vi "DDSSequence_STPrampv1.vi"(6 "Freqeuncy (MHz)":dbl[][](array[numeric]), 7 "Power":dbl[][](array[numeric]), 9 "Channels":T1(ring)=enum."Both channels", 10 "Duration (ms)":dbl[][](array[numeric])) -> (3 "appended instruction string":string="dds reset\rdcp spi:CFR2=0x1000080\rdcp spi:STP0=0x418937\rdcp wait::BNC_IN_A_RISING\rdcp update:u\rdcp spi:STP0=0x339D00002CCCCCCD\rdcp wait:406h:\rdcp update:u\r\rdcp spi:STP0=0x336400002CDBB1CE\rdcp wait:406h:\rdcp update:u\r\rdcp spi:STP0=0x332A00002CEA96CF\rdcp wait:406h:\rdcp update:u\r\rdcp spi:STP0=0x32F100002CF97BD0\rdcp wait:406h:\rdcp update:u\r\rdcp spi:STP0=0x32B800002D0860D1\rdcp wait:406h:\rdcp update:u\r\rdcp spi:STP0=0x327E00002D1745D1\rdcp wait:406h:\rdcp update:u\r\rdcp spi:STP0=0x324500002D262AD2\rdcp wait:406h:\rdcp update:u\r\rdcp spi:STP0=0x320C00002D350FD3\rdcp wait:406h:\rdcp update:u\r\rdcp spi:STP0=0x31D200002D43F4D4\rdcp wait:406h:\rdcp update:u\r\rdcp spi:STP0=0x319900002D52D9D5\rdcp wait:406h:\rdcp update:u\r\rdcp spi:STP0=0x315F00002D61BED6\rdcp wait:406h:\rdcp update:u\r\rdcp spi:STP0=0x312600002D70A3D7\rdcp wait:406h:\rdcp update:u\r\rdcp spi:STP0=0x30ED00002D7F88D8\rdcp wait:406h:\rdcp update:u\r\rdcp spi:STP0=0x30B300002D8E6DD9\rdcp wait:406h:\rdcp update:u\r\rdcp spi:STP0=0x307A00002D9D52DA\rdcp wait:406h:\rdcp update:u\r\rdcp spi:STP0=0x304100002DAC37DB\rdcp wait:406h:\rdcp update:u\r\rdcp spi:STP0=0x300700002DBB1CDC\rdcp wait:406h:\rdcp update:u\r\rdcp spi:STP0=0x2FCE00002DCA01DD\rdcp wait:406h:\rdcp update:u\r\rdcp spi:STP0=0x2F9500002DD8E6DE\rdcp wait:406h:\rdcp update:u\r\rdcp spi:STP0=0x2F5B00002DE7CBDE\rdcp wait:406h:\rdcp update:u\r\rdcp spi:STP0=0x2F4F00002DF6B0DF\rdcp wait:406h:\rdcp update:u\r\rdcp spi:STP0=0x2F4300002E0595E0\rdcp wait:406h:\rdcp update:u\r\rdcp spi:STP0=0x2F3700002E147AE1\rdcp wait:406h:\rdcp update:u\r\rdcp spi:STP0=0x2F2A00002E235FE2\rdcp wait:406h:\rdcp update:u\r\rdcp spi:STP0=0x2F1E00002E3244E3\rdcp wait:406h:\rdcp update:u\r\rdcp spi:STP0=0x2F1200002E4129E4\rdcp wait:406h:\rdcp update:u\r\rdcp spi:STP0=0x2F0500002E500EE5\rdcp wait:406h:\rdcp update:u\r\rdcp spi:STP0=0x2EF900002E5EF3E6\rdcp wait:406h:\rdcp update:u\r\rdcp spi:STP0=0x2EED00002E6DD8E7\rdcp wait:406h:\rdcp update:u\r\rdcp spi:STP0=0x2EE100002E7CBDE8\rdcp wait:406h:\rdcp update:u\r\rdcp spi:STP0=0x2ED400002E8BA2E9\rdcp wait:406h:\rdcp update:u\r\rdcp spi:STP0=0x2EC800002E9A87EA\rdcp wait:406h:\rdcp update:u\r\rdcp spi:STP0=0x2EBC00002EA96CEB\rdcp wait:406h:\rdcp update:u\r\rdcp spi:STP0=0x2EAF00002EB851EC\rdcp wait:406h:\rdcp update:u\r\rdcp spi:STP0=0x2EA300002EC736EC\rdcp wait:406h:\rdcp update:u\r\rdcp spi:STP0=0x2E9700002ED61BED\rdcp wait:406h:\rdcp update:u\r\rdcp spi:STP0=0x2E8B00002EE500EE\rdcp wait:406h:\rdcp update:u\r\rdcp spi:STP0=0x2E7E00002EF3E5EF\rdcp wait:406h:\rdcp update:u\r\rdcp spi:STP0=0x2E7200002F02CAF0\rdcp wait:406h:\rdcp update:u\r\rdcp spi:STP0=0x2E6600002F11AFF1\rdcp wait:406h:\rdcp update:u\r\rdcp spi:STP0=0x2E5900002F2094F2\rdcp wait:406h:\rdcp update:u\r\rdcp spi:STP0=0x2E4D00002F2F79F3\rdcp wait:406h:\rdcp update:u\r\rdcp spi:STP0=0x2E4100002F3E5EF4\rdcp wait:406h:\rdcp update:u\r\rdcp spi:STP0=0x2E3500002F4D43F5\rdcp wait:406h:\rdcp update:u\r\rdcp spi:STP0=0x2E2800002F5C28F6\rdcp wait:406h:\rdcp update:u\r\rdcp spi:STP0=0x2E1C00002F6B0DF7\rdcp wait:406h:\rdcp update:u\r\rdcp spi:STP0=0x2E1000002F79F2F8\rdcp wait:406h:\rdcp update:u\r\rdcp spi:STP0=0x2E0300002F88D7F9\rdcp wait:406h:\rdcp update:u\r\rdcp spi:STP0=0x2DF700002F97BCF9\rdcp wait:406h:\rdcp update:u\r\rdcp spi:STP0=0x2DEB00002FA6A1FA\rdcp wait:406h:\rdcp update:u\r\rdcp spi:STP0=0x2DDF00002FB586FB\rdcp wait:406h:\rdcp update:u\r\rdcp spi:STP0=0x2DD200002FC46BFC\rdcp wait:406h:\rdcp update:u\r\rdcp spi:STP0=0x2DC600002FD350FD\rdcp wait:406h:\rdcp update:u\r\rdcp spi:STP0=0x2DBA00002FE235FE\rdcp wait:406h:\rdcp update:u\r\rdcp spi:STP0=0x2DAD00002FF11AFF\rdcp wait:406h:\rdcp update:u\r\rdcp spi:STP0=0x2DA1000030000000\rdcp wait:406h:\rdcp update:u\r\rdcp spi:STP0=0x2D950000300EE501\rdcp wait:406h:\rdcp update:u\r\rdcp spi:STP0=0x2D890000301DCA02\rdcp wait:406h:\rdcp update:u\r\rdcp spi:STP0=0x2D7C0000302CAF03\rdcp wait:406h:\rdcp update:u\r\rdcp spi:STP0=0x2D700000303B9404\rdcp wait:406h:\rdcp update:u\r\rdcp spi:STP0=0x2D680000304A7905\rdcp wait:406h:\rdcp update:u\r\rdcp spi:STP0=0x2D60000030595E06\rdcp wait:406h:\rdcp update:u\r\rdcp spi:STP0=0x2D57000030684307\rdcp wait:406h:\rdcp update:u\r\rdcp spi:STP0=0x2D4F000030772807\rdcp wait:406h:\rdcp update:u\r\rdcp spi:STP0=0x2D47000030860D08\rdcp wait:406h:\rdcp update:u\r\rdcp spi:STP0=0x2D3F00003094F209\rdcp wait:406h:\rdcp update:u\r\rdcp spi:STP0=0x2D37000030A3D70A\rdcp wait:406h:\rdcp update:u\r\rdcp spi:STP0=0x2D2E000030B2BC0B\rdcp wait:406h:\rdcp update:u\r\rdcp spi:STP0=0x2D26000030C1A10C\rdcp wait:406h:\rdcp update:u\r\rdcp spi:STP0=0x2D1E000030D0860D\rdcp wait:406h:\rdcp update:u\r\rdcp spi:STP0=0x2D16000030DF6B0E\rdcp wait:406h:\rdcp update:u\r\rdcp spi:STP0=0x2D0E000030EE500F\rdcp wait:406h:\rdcp update:u\r\rdcp spi:STP0=0x2D05000030FD3510\rdcp wait:406h:\rdcp update:u\r\rdcp spi:STP0=0x2CFD0000310C1A11\rdcp wait:406h:\rdcp update:u\r\rdcp spi:STP0=0x2CF50000311AFF12\rdcp wait:406h:\rdcp update:u\r\rdcp spi:STP0=0x2CED00003129E413\rdcp wait:406h:\rdcp update:u\r\rdcp spi:STP0=0x2CE500003138C914\rdcp wait:406h:\rdcp update:u\r\rdcp spi:STP0=0x2CDC00003147AE14\rdcp wait:406h:\rdcp update:u\r\rdcp spi:STP0=0x2CD4000031569315\rdcp wait:406h:\rdcp update:u\r\rdcp spi:STP0=0x2CCC000031657816\rdcp wait:406h:\rdcp update:u\r\rdcp spi:STP0=0x2CC4000031745D17\rdcp wait:406h:\rdcp update:u\r\rdcp spi:STP0=0x2CBC000031834218\rdcp wait:406h:\rdcp update:u\r\rdcp spi:STP0=0x2CB4000031922719\rdcp wait:406h:\rdcp update:u\r\rdcp spi:STP0=0x2CAB000031A10C1A\rdcp wait:406h:\rdcp update:u\r\rdcp spi:STP0=0x2CA3000031AFF11B\rdcp wait:406h:\rdcp update:u\r\rdcp spi:STP0=0x2C9B000031BED61C\rdcp wait:406h:\rdcp update:u\r\rdcp spi:STP0=0x2C93000031CDBB1D\rdcp wait:406h:\rdcp update:u\r\rdcp spi:STP0=0x2C8B000031DCA01E\rdcp wait:406h:\rdcp update:u\r\rdcp spi:STP0=0x2C82000031EB851F\rdcp wait:406h:\rdcp update:u\r\rdcp spi:STP0=0x2C7A000031FA6A20\rdcp wait:406h:\rdcp update:u\r\rdcp spi:STP0=0x2C72000032094F21\rdcp wait:406h:\rdcp update:u\r\rdcp spi:STP0=0x2C6A000032183422\rdcp wait:406h:\rdcp update:u\r\rdcp spi:STP0=0x2C62000032271922\rdcp wait:406h:\rdcp update:u\r\rdcp spi:STP0=0x2C5900003235FE23\rdcp wait:406h:\rdcp update:u\r\rdcp spi:STP0=0x2C5100003244E324\rdcp wait:406h:\rdcp update:u\r\rdcp spi:STP0=0x2C4900003253C825\rdcp wait:406h:\rdcp update:u\r\rdcp spi:STP0=0x2C4100003262AD26\rdcp wait:406h:\rdcp update:u\r\rdcp spi:STP0=0x2C39000032719227\rdcp wait:406h:\rdcp update:u\r\rdcp spi:STP0=0x2C30000032807728\rdcp wait:406h:\rdcp update:u\r\rdcp spi:STP0=0x2C280000328F5C29\rdcp wait:406h:\rdcp update:u\r\rdcp spi:STP0=0x2C1C0000329E412A\rdcp wait:406h:\rdcp update:u\r\rdcp spi:STP0=0x2C10000032AD262B\rdcp wait:406h:\rdcp update:u\r\rdcp spi:STP0=0x2C03000032BC0B2C\rdcp wait:406h:\rdcp update:u\r\rdcp spi:STP0=0x2BF7000032CAF02D\rdcp wait:406h:\rdcp update:u\r\rdcp spi:STP0=0x2BEB000032D9D52E\rdcp wait:406h:\rdcp update:u\r\rdcp spi:STP0=0x2BDF000032E8BA2F\rdcp wait:406h:\rdcp update:u\r\rdcp spi:STP0=0x2BD2000032F79F2F\rdcp wait:406h:\rdcp update:u\r\rdcp spi:STP0=0x2BC6000033068430\rdcp wait:406h:\rdcp update:u\r\rdcp spi:STP0=0x2BBA000033156931\rdcp wait:406h:\rdcp update:u\r\rdcp spi:STP0=0x2BAD000033244E32\rdcp wait:406h:\rdcp update:u\r\rdcp spi:STP0=0x2BA1000033333333\rdcp wait:406h:\rdcp update:u\r\rdcp spi:STP0=0x2B95000033421834\rdcp wait:406h:\rdcp update:u\r\rdcp spi:STP0=0x2B8900003350FD35\rdcp wait:406h:\rdcp update:u\r\rdcp spi:STP0=0x2B7C0000335FE236\rdcp wait:406h:\rdcp update:u\r\rdcp spi:STP0=0x2B700000336EC737\rdcp wait:406h:\rdcp update:u\r\rdcp spi:STP0=0x2B640000337DAC38\rdcp wait:406h:\rdcp update:u\r\rdcp spi:STP0=0x2B570000338C9139\rdcp wait:406h:\rdcp update:u\r\rdcp spi:STP0=0x2B4B0000339B763A\rdcp wait:406h:\rdcp update:u\r\rdcp spi:STP0=0x2B3F000033AA5B3B\rdcp wait:406h:\rdcp update:u\r\rdcp spi:STP0=0x2B33000033B9403C\rdcp wait:406h:\rdcp update:u\r\rdcp spi:STP0=0x2B26000033C8253D\rdcp wait:406h:\rdcp update:u\r\rdcp spi:STP0=0x2B1A000033D70A3D\rdcp wait:406h:\rdcp update:u\r\rdcp spi:STP0=0x2B0E000033E5EF3E\rdcp wait:406h:\rdcp update:u\r\rdcp spi:STP0=0x2B01000033F4D43F\rdcp wait:406h:\rdcp update:u\r\rdcp spi:STP0=0x2AF500003403B940\rdcp wait:406h:\rdcp update:u\r\rdcp spi:STP0=0x2AE9000034129E41\rdcp wait:406h:\rdcp update:u\r\rdcp spi:STP0=0x2ADD000034218342\rdcp wait:406h:\rdcp update:u\r\rdcp spi:STP0=0x2AD0000034306843\rdcp wait:406h:\rdcp update:u\r\rdcp spi:STP0=0x2AC40000343F4D44\rdcp wait:406h:\rdcp update:u\r\rdcp spi:STP0=0x2AB80000344E3245\rdcp wait:406h:\rdcp update:u\r\rdcp spi:STP0=0x2AAB0000345D1746\rdcp wait:406h:\rdcp update:u\r\rdcp spi:STP0=0x2A9F0000346BFC47\rdcp wait:406h:\rdcp update:u\r\rdcp spi:STP0=0x2A930000347AE148\rdcp wait:406h:\rdcp update:u\r\rdcp spi:STP0=0x2A8700003489C649\rdcp wait:406h:\rdcp update:u\r\rdcp spi:STP0=0x2A7A00003498AB4A\rdcp wait:406h:\rdcp update:u\r\rdcp spi:STP0=0x2A6E000034A7904A\rdcp wait:406h:\rdcp update:u\r\rdcp spi:STP0=0x2A62000034B6754B\rdcp wait:406h:\rdcp update:u\r\rdcp spi:STP0=0x2A55000034C55A4C\rdcp wait:406h:\rdcp update:u\r\rdcp spi:STP0=0x2A49000034D43F4D\rdcp wait:406h:\rdcp update:u\r\rdcp spi:STP0=0x2A3D000034E3244E\rdcp wait:406h:\rdcp update:u\r\rdcp spi:STP0=0x2A28000034F2094F\rdcp wait:406h:\rdcp update:u\r\rdcp spi:STP0=0x2A1400003500EE50\rdcp wait:406h:\rdcp update:u\r\rdcp spi:STP0=0x29FF0000350FD351\rdcp wait:406h:\rdcp update:u\r\rdcp spi:STP0=0x29EB0000351EB852\rdcp wait:406h:\rdcp update:u\r\rdcp spi:STP0=0x29D60000352D9D53\rdcp wait:406h:\rdcp update:u\r\rdcp spi:STP0=0x29C20000353C8254\rdcp wait:406h:\rdcp update:u\r\rdcp spi:STP0=0x29AD0000354B6755\rdcp wait:406h:\rdcp update:u\r\rdcp spi:STP0=0x29990000355A4C56\rdcp wait:406h:\rdcp update:u\r\rdcp spi:STP0=0x2984000035693157\rdcp wait:406h:\rdcp update:u\r\rdcp spi:STP0=0x2970000035781658\rdcp wait:406h:\rdcp update:u\r\rdcp spi:STP0=0x295C00003586FB58\rdcp wait:406h:\rdcp update:u\r\rdcp spi:STP0=0x294700003595E059\rdcp wait:406h:\rdcp update:u\r\rdcp spi:STP0=0x2933000035A4C55A\rdcp wait:406h:\rdcp update:u\r\rdcp spi:STP0=0x291E000035B3AA5B\rdcp wait:406h:\rdcp update:u\r\rdcp spi:STP0=0x290A000035C28F5C\rdcp wait:406h:\rdcp update:u\r\rdcp spi:STP0=0x28F5000035D1745D\rdcp wait:406h:\rdcp update:u\r\rdcp spi:STP0=0x28E1000035E0595E\rdcp wait:406h:\rdcp update:u\r\rdcp spi:STP0=0x28CC000035EF3E5F\rdcp wait:406h:\rdcp update:u\r\rdcp spi:STP0=0x28B8000035FE2360\rdcp wait:406h:\rdcp update:u\r\rdcp spi:STP0=0x28A30000360D0861\rdcp wait:406h:\rdcp update:u\r\rdcp spi:STP0=0x288F0000361BED62\rdcp wait:406h:\rdcp update:u\r\rdcp spi:STP0=0x287A0000362AD263\rdcp wait:406h:\rdcp update:u\r\rdcp spi:STP0=0x286600003639B764\rdcp wait:406h:\rdcp update:u\r\rdcp spi:STP0=0x2851000036489C65\rdcp wait:406h:\rdcp update:u\r\rdcp spi:STP0=0x283D000036578165\rdcp wait:406h:\rdcp update:u\r\rdcp spi:STP0=0x2828000036666666\rdcp wait:406h:\rdcp update:u\r\rdcp spi:STP0=0x2814000036754B67\rdcp wait:406h:\rdcp update:u\r\rdcp spi:STP0=0x27FF000036843068\rdcp wait:406h:\rdcp update:u\r\rdcp spi:STP0=0x27EB000036931569\rdcp wait:406h:\rdcp update:u\r\rdcp spi:STP0=0x27D6000036A1FA6A\rdcp wait:406h:\rdcp update:u\r\rdcp spi:STP0=0x27C2000036B0DF6B\rdcp wait:406h:\rdcp update:u\r\rdcp spi:STP0=0x27AD000036BFC46C\rdcp wait:406h:\rdcp update:u\r\rdcp spi:STP0=0x2799000036CEA96D\rdcp wait:406h:\rdcp update:u\r\rdcp spi:STP0=0x2785000036DD8E6E\rdcp wait:406h:\rdcp update:u\r\rdcp spi:STP0=0x2770000036EC736F\rdcp wait:406h:\rdcp update:u\r\rdcp spi:STP0=0x275C000036FB5870\rdcp wait:406h:\rdcp update:u\r\rdcp spi:STP0=0x27470000370A3D71\rdcp wait:406h:\rdcp update:u\r\rdcp spi:STP0=0x2733000037192272\rdcp wait:406h:\rdcp update:u\r\rdcp spi:STP0=0x271E000037280773\rdcp wait:406h:\rdcp update:u\r\rdcp spi:STP0=0x270A00003736EC73\rdcp wait:406h:\rdcp update:u\r\rdcp spi:STP0=0x26FD00003745D174\rdcp wait:406h:\rdcp update:u\r\rdcp spi:STP0=0x26F100003754B675\rdcp wait:406h:\rdcp update:u\r\rdcp spi:STP0=0x26E5000037639B76\rdcp wait:406h:\rdcp update:u\r\rdcp spi:STP0=0x26D8000037728077\rdcp wait:406h:\rdcp update:u\r\rdcp spi:STP0=0x26CC000037816578\rdcp wait:406h:\rdcp update:u\r\rdcp spi:STP0=0x26C0000037904A79\rdcp wait:406h:\rdcp update:u\r\rdcp spi:STP0=0x26B40000379F2F7A\rdcp wait:406h:\rdcp update:u\r\rdcp spi:STP0=0x26A7000037AE147B\rdcp wait:406h:\rdcp update:u\r\rdcp spi:STP0=0x269B000037BCF97C\rdcp wait:406h:\rdcp update:u\r\rdcp spi:STP0=0x268F000037CBDE7D\rdcp wait:406h:\rdcp update:u\r\rdcp spi:STP0=0x2682000037DAC37E\rdcp wait:406h:\rdcp update:u\r\rdcp spi:STP0=0x2676000037E9A87F\rdcp wait:406h:\rdcp update:u\r\rdcp spi:STP0=0x266A000037F88D80\rdcp wait:406h:\rdcp update:u\r\rdcp spi:STP0=0x265E000038077280\rdcp wait:406h:\rdcp update:u\r\rdcp spi:STP0=0x2651000038165781\rdcp wait:406h:\rdcp update:u\r\rdcp spi:STP0=0x2645000038253C82\rdcp wait:406h:\rdcp update:u\r\rdcp spi:STP0=0x2639000038342183\rdcp wait:406h:\rdcp update:u\r\rdcp spi:STP0=0x262C000038430684\rdcp wait:406h:\rdcp update:u\r\rdcp spi:STP0=0x262000003851EB85\rdcp wait:406h:\rdcp update:u\r\rdcp spi:STP0=0x261400003860D086\rdcp wait:406h:\rdcp update:u\r\rdcp spi:STP0=0x26080000386FB587\rdcp wait:406h:\rdcp update:u\r\rdcp spi:STP0=0x25FB0000387E9A88\rdcp wait:406h:\rdcp update:u\r\rdcp spi:STP0=0x25EF0000388D7F89\rdcp wait:406h:\rdcp update:u\r\rdcp spi:STP0=0x25E30000389C648A\rdcp wait:406h:\rdcp update:u\r\rdcp spi:STP0=0x25D6000038AB498B\rdcp wait:406h:\rdcp update:u\r\rdcp spi:STP0=0x25CA000038BA2E8C\rdcp wait:406h:\rdcp update:u\r\rdcp spi:STP0=0x25BE000038C9138D\rdcp wait:406h:\rdcp update:u\r\rdcp spi:STP0=0x25B2000038D7F88D\rdcp wait:406h:\rdcp update:u\r\rdcp spi:STP0=0x25A5000038E6DD8E\rdcp wait:406h:\rdcp update:u\r\rdcp spi:STP0=0x2599000038F5C28F\rdcp wait:406h:\rdcp update:u\r\rdcp spi:STP0=0x258D00003904A790\rdcp wait:406h:\rdcp update:u\r\rdcp spi:STP0=0x2580000039138C91\rdcp wait:406h:\rdcp update:u\r\rdcp spi:STP0=0x2574000039227192\rdcp wait:406h:\rdcp update:u\r\rdcp spi:STP0=0x2568000039315693\rdcp wait:406h:\rdcp update:u\r\rdcp spi:STP0=0x255C000039403B94\rdcp wait:406h:\rdcp update:u\r\rdcp spi:STP0=0x254F0000394F2095\rdcp wait:406h:\rdcp update:u\r\rdcp spi:STP0=0x25430000395E0596\rdcp wait:406h:\rdcp update:u\r\rdcp spi:STP0=0x25370000396CEA97\rdcp wait:406h:\rdcp update:u\r\rdcp spi:STP0=0x252A0000397BCF98\rdcp wait:406h:\rdcp update:u\r\rdcp spi:STP0=0x251E0000398AB499\rdcp wait:406h:\rdcp update:u\r\rdcp spi:STP0=0x251A00003999999A\rdcp wait:406h:\rdcp update:u\r\rdcp spi:STP0=0x2516000039A87E9B\rdcp wait:406h:\rdcp update:u\r\rdcp spi:STP0=0x2512000039B7639B\rdcp wait:406h:\rdcp update:u\r\rdcp spi:STP0=0x250E000039C6489C\rdcp wait:406h:\rdcp update:u\r\rdcp spi:STP0=0x250A000039D52D9D\rdcp wait:406h:\rdcp update:u\r\rdcp spi:STP0=0x2506000039E4129E\rdcp wait:406h:\rdcp update:u\r\rdcp spi:STP0=0x2501000039F2F79F\rdcp wait:406h:\rdcp update:u\r\rdcp spi:STP0=0x24FD00003A01DCA0\rdcp wait:406h:\rdcp update:u\r\rdcp spi:STP0=0x24F900003A10C1A1\rdcp wait:406h:\rdcp update:u\r\rdcp spi:STP0=0x24F500003A1FA6A2\rdcp wait:406h:\rdcp update:u\r\rdcp spi:STP0=0x24F100003A2E8BA3\rdcp wait:406h:\rdcp update:u\r\rdcp spi:STP0=0x24ED00003A3D70A4\rdcp wait:406h:\rdcp update:u\r\rdcp spi:STP0=0x24E900003A4C55A5\rdcp wait:406h:\rdcp update:u\r\rdcp spi:STP0=0x24E500003A5B3AA6\rdcp wait:406h:\rdcp update:u\r\rdcp spi:STP0=0x24E100003A6A1FA7\rdcp wait:406h:\rdcp update:u\r\rdcp spi:STP0=0x24DD00003A7904A8\rdcp wait:406h:\rdcp update:u\r\rdcp spi:STP0=0x24D900003A87E9A8\rdcp wait:406h:\rdcp update:u\r\rdcp spi:STP0=0x24D400003A96CEA9\rdcp wait:406h:\rdcp update:u\r\rdcp spi:STP0=0x24D000003AA5B3AA\rdcp wait:406h:\rdcp update:u\r\rdcp spi:STP0=0x24CC00003AB498AB\rdcp wait:406h:\rdcp update:u\r\rdcp spi:STP0=0x24C800003AC37DAC\rdcp wait:406h:\rdcp update:u\r\rdcp spi:STP0=0x24C400003AD262AD\rdcp wait:406h:\rdcp update:u\r\rdcp spi:STP0=0x24C000003AE147AE\rdcp wait:406h:\rdcp update:u\r\rdcp spi:STP0=0x24BC00003AF02CAF\rdcp wait:406h:\rdcp update:u\r\rdcp spi:STP0=0x24B800003AFF11B0\rdcp wait:406h:\rdcp update:u\r\rdcp spi:STP0=0x24B400003B0DF6B1\rdcp wait:406h:\rdcp update:u\r\rdcp spi:STP0=0x24B000003B1CDBB2\rdcp wait:406h:\rdcp update:u\r\rdcp spi:STP0=0x24AB00003B2BC0B3\rdcp wait:406h:\rdcp update:u\r\rdcp spi:STP0=0x24A700003B3AA5B4\rdcp wait:406h:\rdcp update:u\r\rdcp spi:STP0=0x24A300003B498AB5\rdcp wait:406h:\rdcp update:u\r\rdcp spi:STP0=0x249F00003B586FB6\rdcp wait:406h:\rdcp update:u\r\rdcp spi:STP0=0x249B00003B6754B6\rdcp wait:406h:\rdcp update:u\r\rdcp spi:STP0=0x249700003B7639B7\rdcp wait:406h:\rdcp update:u\r\rdcp spi:STP0=0x249300003B851EB8\rdcp wait:406h:\rdcp update:u\r\rdcp spi:STP0=0x248F00003B9403B9\rdcp wait:406h:\rdcp update:u\r\rdcp spi:STP0=0x248B00003BA2E8BA\rdcp wait:406h:\rdcp update:u\r\rdcp spi:STP0=0x248700003BB1CDBB\rdcp wait:406h:\rdcp update:u\r\rdcp spi:STP0=0x248300003BC0B2BC\rdcp wait:406h:\rdcp update:u\r\rdcp spi:STP0=0x247E00003BCF97BD\rdcp wait:406h:\rdcp update:u\r\rdcp spi:STP0=0x247A00003BDE7CBE\rdcp wait:406h:\rdcp update:u\r\rdcp spi:STP0=0x247E00003BED61BF\rdcp wait:406h:\rdcp update:u\r\rdcp spi:STP0=0x248300003BFC46C0\rdcp wait:406h:\rdcp update:u\r\rdcp spi:STP0=0x248700003C0B2BC1\rdcp wait:406h:\rdcp update:u\r\rdcp spi:STP0=0x248B00003C1A10C2\rdcp wait:406h:\rdcp update:u\r\rdcp spi:STP0=0x248F00003C28F5C3\rdcp wait:406h:\rdcp update:u\r\rdcp spi:STP0=0x249300003C37DAC3\rdcp wait:406h:\rdcp update:u\r\rdcp spi:STP0=0x249700003C46BFC4\rdcp wait:406h:\rdcp update:u\r\rdcp spi:STP0=0x249B00003C55A4C5\rdcp wait:406h:\rdcp update:u\r\rdcp spi:STP0=0x249F00003C6489C6\rdcp wait:406h:\rdcp update:u\r\rdcp spi:STP0=0x24A300003C736EC7\rdcp wait:406h:\rdcp update:u\r\rdcp spi:STP0=0x24A700003C8253C8\rdcp wait:406h:\rdcp update:u\r\rdcp spi:STP0=0x24AB00003C9138C9\rdcp wait:406h:\rdcp update:u\r\rdcp spi:STP0=0x24B000003CA01DCA\rdcp wait:406h:\rdcp update:u\r\rdcp spi:STP0=0x24B400003CAF02CB\rdcp wait:406h:\rdcp update:u\r\rdcp spi:STP0=0x24B800003CBDE7CC\rdcp wait:406h:\rdcp update:u\r\rdcp spi:STP0=0x24BC00003CCCCCCD\rdcp wait:406h:\rdcp update:u\r\rdcp spi:STP0=0x24C000003CDBB1CE\rdcp wait:406h:\rdcp update:u\r\rdcp spi:STP0=0x24C400003CEA96CF\rdcp wait:406h:\rdcp update:u\r\rdcp spi:STP0=0x24C800003CF97BD0\rdcp wait:406h:\rdcp update:u\r\rdcp spi:STP0=0x24CC00003D0860D1\rdcp wait:406h:\rdcp update:u\r\rdcp spi:STP0=0x24D000003D1745D1\rdcp wait:406h:\rdcp update:u\r\rdcp spi:STP0=0x24D400003D262AD2\rdcp wait:406h:\rdcp update:u\r\rdcp spi:STP0=0x24D900003D350FD3\rdcp wait:406h:\rdcp update:u\r\rdcp spi:STP0=0x24DD00003D43F4D4\rdcp wait:406h:\rdcp update:u\r\rdcp spi:STP0=0x24E100003D52D9D5\rdcp wait:406h:\rdcp update:u\r\rdcp spi:STP0=0x24E500003D61BED6\rdcp wait:406h:\rdcp update:u\r\rdcp spi:STP0=0x24E900003D70A3D7\rdcp wait:406h:\rdcp update:u\r\rdcp spi:STP0=0x24ED00003D7F88D8\rdcp wait:406h:\rdcp update:u\r\rdcp spi:STP0=0x24F100003D8E6DD9\rdcp wait:406h:\rdcp update:u\r\rdcp spi:STP0=0x24F500003D9D52DA\rdcp wait:406h:\rdcp update:u\r\rdcp spi:STP0=0x24F900003DAC37DB\rdcp wait:406h:\rdcp update:u\r\rdcp spi:STP0=0x24FD00003DBB1CDC\rdcp wait:406h:\rdcp update:u\r\rdcp spi:STP0=0x250100003DCA01DD\rdcp wait:406h:\rdcp update:u\r\rdcp spi:STP0=0x250600003DD8E6DE\rdcp wait:406h:\rdcp update:u\r\rdcp spi:STP0=0x250A00003DE7CBDE\rdcp wait:406h:\rdcp update:u\r\rdcp spi:STP0=0x250E00003DF6B0DF\rdcp wait:406h:\rdcp update:u\r\rdcp spi:STP0=0x251200003E0595E0\rdcp wait:406h:\rdcp update:u\r\rdcp spi:STP0=0x251600003E147AE1\rdcp wait:406h:\rdcp update:u\r\rdcp spi:STP0=0x251A00003E235FE2\rdcp wait:406h:\rdcp update:u\r\rdcp spi:STP0=0x251E00003E3244E3\rdcp wait:406h:\rdcp update:u\r\rdcp spi:STP0=0x252A00003E4129E4\rdcp wait:406h:\rdcp update:u\r\rdcp spi:STP0=0x253700003E500EE5\rdcp wait:406h:\rdcp update:u\r\rdcp spi:STP0=0x254300003E5EF3E6\rdcp wait:406h:\rdcp update:u\r\rdcp spi:STP0=0x254F00003E6DD8E7\rdcp wait:406h:\rdcp update:u\r\rdcp spi:STP0=0x255C00003E7CBDE8\rdcp wait:406h:\rdcp update:u\r\rdcp spi:STP0=0x256800003E8BA2E9\rdcp wait:406h:\rdcp update:u\r\rdcp spi:STP0=0x257400003E9A87EA\rdcp wait:406h:\rdcp update:u\r\rdcp spi:STP0=0x258000003EA96CEB\rdcp wait:406h:\rdcp update:u\r\rdcp spi:STP0=0x258D00003EB851EC\rdcp wait:406h:\rdcp update:u\r\rdcp spi:STP0=0x259900003EC736EC\rdcp wait:406h:\rdcp update:u\r\rdcp spi:STP0=0x25A500003ED61BED\rdcp wait:406h:\rdcp update:u\r\rdcp spi:STP0=0x25B200003EE500EE\rdcp wait:406h:\rdcp update:u\r\rdcp spi:STP0=0x25BE00003EF3E5EF\rdcp wait:406h:\rdcp update:u\r\rdcp spi:STP0=0x25CA00003F02CAF0\rdcp wait:406h:\rdcp update:u\r\rdcp spi:STP0=0x25D600003F11AFF1\rdcp wait:406h:\rdcp update:u\r\rdcp spi:STP0=0x25E300003F2094F2\rdcp wait:406h:\rdcp update:u\r\rdcp spi:STP0=0x25EF00003F2F79F3\rdcp wait:406h:\rdcp update:u\r\rdcp spi:STP0=0x25FB00003F3E5EF4\rdcp wait:406h:\rdcp update:u\r\rdcp spi:STP0=0x260800003F4D43F5\rdcp wait:406h:\rdcp update:u\r\rdcp spi:STP0=0x261400003F5C28F6\rdcp wait:406h:\rdcp update:u\r\rdcp spi:STP0=0x262000003F6B0DF7\rdcp wait:406h:\rdcp update:u\r\rdcp spi:STP0=0x262C00003F79F2F8\rdcp wait:406h:\rdcp update:u\r\rdcp spi:STP0=0x263900003F88D7F9\rdcp wait:406h:\rdcp update:u\r\rdcp spi:STP0=0x264500003F97BCF9\rdcp wait:406h:\rdcp update:u\r\rdcp spi:STP0=0x265100003FA6A1FA\rdcp wait:406h:\rdcp update:u\r\rdcp spi:STP0=0x265E00003FB586FB\rdcp wait:406h:\rdcp update:u\r\rdcp spi:STP0=0x266A00003FC46BFC\rdcp wait:406h:\rdcp update:u\r\rdcp spi:STP0=0x267600003FD350FD\rdcp wait:406h:\rdcp update:u\r\rdcp spi:STP0=0x268200003FE235FE\rdcp wait:406h:\rdcp update:u\r\rdcp spi:STP0=0x268F00003FF11AFF\rdcp wait:406h:\rdcp update:u\r\rdcp spi:STP0=0x269B000040000000\rdcp wait:406h:\rdcp update:u\r\rdcp spi:STP0=0x26A70000400EE501\rdcp wait:406h:\rdcp update:u\r\rdcp spi:STP0=0x26B40000401DCA02\rdcp wait:406h:\rdcp update:u\r\rdcp spi:STP0=0x26C00000402CAF03\rdcp wait:406h:\rdcp update:u\r\rdcp spi:STP0=0x26CC0000403B9404\rdcp wait:406h:\rdcp update:u\r\rdcp spi:STP0=0x26D80000404A7905\rdcp wait:406h:\rdcp update:u\r\rdcp spi:STP0=0x26E5000040595E06\rdcp wait:406h:\rdcp update:u\r\rdcp spi:STP0=0x26F1000040684307\rdcp wait:406h:\rdcp update:u\r\rdcp spi:STP0=0x26FD000040772807\rdcp wait:406h:\rdcp update:u\r\rdcp spi:STP0=0x270A000040860D08\rdcp wait:406h:\rdcp update:u\r\rdcp spi:STP0=0x271A00004094F209\rdcp wait:406h:\rdcp update:u\r\rdcp spi:STP0=0x272A000040A3D70A\rdcp wait:406h:\rdcp update:u\r\rdcp spi:STP0=0x273B000040B2BC0B\rdcp wait:406h:\rdcp update:u\r\rdcp spi:STP0=0x274B000040C1A10C\rdcp wait:406h:\rdcp update:u\r\rdcp spi:STP0=0x275C000040D0860D\rdcp wait:406h:\rdcp update:u\r\rdcp spi:STP0=0x276C000040DF6B0E\rdcp wait:406h:\rdcp update:u\r\rdcp spi:STP0=0x277C000040EE500F\rdcp wait:406h:\rdcp update:u\r\rdcp spi:STP0=0x278D000040FD3510\rdcp wait:406h:\rdcp update:u\r\rdcp spi:STP0=0x279D0000410C1A11\rdcp wait:406h:\rdcp update:u\r\rdcp spi:STP0=0x27AD0000411AFF12\rdcp wait:406h:\rdcp update:u\r\rdcp spi:STP0=0x27BE00004129E413\rdcp wait:406h:\rdcp update:u\r\rdcp spi:STP0=0x27CE00004138C914\rdcp wait:406h:\rdcp update:u\r\rdcp spi:STP0=0x27DF00004147AE14\rdcp wait:406h:\rdcp update:u\r\rdcp spi:STP0=0x27EF000041569315\rdcp wait:406h:\rdcp update:u\r\rdcp spi:STP0=0x27FF000041657816\rdcp wait:406h:\rdcp update:u\r\rdcp spi:STP0=0x2810000041745D17\rdcp wait:406h:\rdcp update:u\r\rdcp spi:STP0=0x2820000041834218\rdcp wait:406h:\rdcp update:u\r\rdcp spi:STP0=0x2831000041922719\rdcp wait:406h:\rdcp update:u\r\rdcp spi:STP0=0x2841000041A10C1A\rdcp wait:406h:\rdcp update:u\r\rdcp spi:STP0=0x2851000041AFF11B\rdcp wait:406h:\rdcp update:u\r\rdcp spi:STP0=0x2862000041BED61C\rdcp wait:406h:\rdcp update:u\r\rdcp spi:STP0=0x2872000041CDBB1D\rdcp wait:406h:\rdcp update:u\r\rdcp spi:STP0=0x2882000041DCA01E\rdcp wait:406h:\rdcp update:u\r\rdcp spi:STP0=0x2893000041EB851F\rdcp wait:406h:\rdcp update:u\r\rdcp spi:STP0=0x28A3000041FA6A20\rdcp wait:406h:\rdcp update:u\r\rdcp spi:STP0=0x28B4000042094F21\rdcp wait:406h:\rdcp update:u\r\rdcp spi:STP0=0x28C4000042183422\rdcp wait:406h:\rdcp update:u\r\rdcp spi:STP0=0x28D4000042271922\rdcp wait:406h:\rdcp update:u\r\rdcp spi:STP0=0x28E500004235FE23\rdcp wait:406h:\rdcp update:u\r\rdcp spi:STP0=0x28F500004244E324\rdcp wait:406h:\rdcp update:u\r\rdcp spi:STP0=0x290600004253C825\rdcp wait:406h:\rdcp update:u\r\rdcp spi:STP0=0x291600004262AD26\rdcp wait:406h:\rdcp update:u\r\rdcp spi:STP0=0x2926000042719227\rdcp wait:406h:\rdcp update:u\r\rdcp spi:STP0=0x2937000042807728\rdcp wait:406h:\rdcp update:u\r\rdcp spi:STP0=0x29470000428F5C29\rdcp wait:406h:\rdcp update:u\r\rdcp spi:STP0=0x29570000429E412A\rdcp wait:406h:\rdcp update:u\r\rdcp spi:STP0=0x2968000042AD262B\rdcp wait:406h:\rdcp update:u\r\rdcp spi:STP0=0x2978000042BC0B2C\rdcp wait:406h:\rdcp update:u\r\rdcp spi:STP0=0x2989000042CAF02D\rdcp wait:406h:\rdcp update:u\r\rdcp spi:STP0=0x2999000042D9D52E\rdcp wait:406h:\rdcp update:u\r\rdcp spi:STP0=0x29C2000042E8BA2F\rdcp wait:406h:\rdcp update:u\r\rdcp spi:STP0=0x29EB000042F79F2F\rdcp wait:406h:\rdcp update:u\r\rdcp spi:STP0=0x2A14000043068430\rdcp wait:406h:\rdcp update:u\r\rdcp spi:STP0=0x2A3D000043156931\rdcp wait:406h:\rdcp update:u\r\rdcp spi:STP0=0x2A66000043244E32\rdcp wait:406h:\rdcp update:u\r\rdcp spi:STP0=0x2A8F000043333333\rdcp wait:406h:\rdcp update:u\r\rdcp spi:STP0=0x2AB8000043421834\rdcp wait:406h:\rdcp update:u\r\rdcp spi:STP0=0x2AE100004350FD35\rdcp wait:406h:\rdcp update:u\r\rdcp spi:STP0=0x2B0A0000435FE236\rdcp wait:406h:\rdcp update:u\r\rdcp spi:STP0=0x2B330000436EC737\rdcp wait:406h:\rdcp update:u\r\rdcp spi:STP0=0x2B5B0000437DAC38\rdcp wait:406h:\rdcp update:u\r\rdcp spi:STP0=0x2B840000438C9139\rdcp wait:406h:\rdcp update:u\r\rdcp spi:STP0=0x2BAD0000439B763A\rdcp wait:406h:\rdcp update:u\r\rdcp spi:STP0=0x2BD6000043AA5B3B\rdcp wait:406h:\rdcp update:u\r\rdcp spi:STP0=0x2BFF000043B9403C\rdcp wait:406h:\rdcp update:u\r\rdcp spi:STP0=0x2C28000043C8253D\rdcp wait:406h:\rdcp update:u\r\rdcp spi:STP0=0x2C51000043D70A3D\rdcp wait:406h:\rdcp update:u\r\rdcp spi:STP0=0x2C7A000043E5EF3E\rdcp wait:406h:\rdcp update:u\r\rdcp spi:STP0=0x2CA3000043F4D43F\rdcp wait:406h:\rdcp update:u\r\rdcp spi:STP0=0x2CCC00004403B940\rdcp wait:406h:\rdcp update:u\r\rdcp spi:STP0=0x2CF5000044129E41\rdcp wait:406h:\rdcp update:u\r\rdcp spi:STP0=0x2D1E000044218342\rdcp wait:406h:\rdcp update:u\r\rdcp spi:STP0=0x2D47000044306843\rdcp wait:406h:\rdcp update:u\r\rdcp spi:STP0=0x2D700000443F4D44\rdcp wait:406h:\rdcp update:u\r\rdcp spi:STP0=0x2D990000444E3245\rdcp wait:406h:\rdcp update:u\r\rdcp spi:STP0=0x2DC20000445D1746\rdcp wait:406h:\rdcp update:u\r\rdcp spi:STP0=0x2DEB0000446BFC47\rdcp wait:406h:\rdcp update:u\r\rdcp spi:STP0=0x2E140000447AE148\rdcp wait:406h:\rdcp update:u\r\rdcp spi:STP0=0x2E3D00004489C649\rdcp wait:406h:\rdcp update:u\r\rdcp spi:STP0=0x2E6600004498AB4A\rdcp wait:406h:\rdcp update:u\r\rdcp spi:STP0=0x2E8F000044A7904A\rdcp wait:406h:\rdcp update:u\r\rdcp spi:STP0=0x2EB8000044B6754B\rdcp wait:406h:\rdcp update:u\r\rdcp spi:STP0=0x2EE1000044C55A4C\rdcp wait:406h:\rdcp update:u\r\rdcp spi:STP0=0x2F0A000044D43F4D\rdcp wait:406h:\rdcp update:u\r\rdcp spi:STP0=0x2F32000044E3244E\rdcp wait:406h:\rdcp update:u\r\rdcp spi:STP0=0x2F5B000044F2094F\rdcp wait:406h:\rdcp update:u\r\rdcp spi:STP0=0x2F8400004500EE50\rdcp wait:406h:\rdcp update:u\r\rdcp spi:STP0=0x2FAD0000450FD351\rdcp wait:406h:\rdcp update:u\r\rdcp spi:STP0=0x2FD60000451EB852\rdcp wait:406h:\rdcp update:u\r\rdcp spi:STP0=0x2FFF0000452D9D53\rdcp wait:406h:\rdcp update:u\r\rdcp spi:STP0=0x30510000453C8254\rdcp wait:406h:\rdcp update:u\r\rdcp spi:STP0=0x30A30000454B6755\rdcp wait:406h:\rdcp update:u\r\rdcp spi:STP0=0x30F50000455A4C56\rdcp wait:406h:\rdcp update:u\r\rdcp spi:STP0=0x3147000045693157\rdcp wait:406h:\rdcp update:u\r\rdcp spi:STP0=0x3199000045781658\rdcp wait:406h:\rdcp update:u\r\rdcp spi:STP0=0x31EB00004586FB58\rdcp wait:406h:\rdcp update:u\r\rdcp spi:STP0=0x323D00004595E059\rdcp wait:406h:\rdcp update:u\r\rdcp spi:STP0=0x328F000045A4C55A\rdcp wait:406h:\rdcp update:u\r\rdcp spi:STP0=0x32E0000045B3AA5B\rdcp wait:406h:\rdcp update:u\r\rdcp spi:STP0=0x3332000045C28F5C\rdcp wait:406h:\rdcp update:u\r\rdcp spi:STP0=0x3384000045D1745D\rdcp wait:406h:\rdcp update:u\r\rdcp spi:STP0=0x33D6000045E0595E\rdcp wait:406h:\rdcp update:u\r\rdcp spi:STP0=0x3428000045EF3E5F\rdcp wait:406h:\rdcp update:u\r\rdcp spi:STP0=0x347A000045FE2360\rdcp wait:406h:\rdcp update:u\r\rdcp spi:STP0=0x34CC0000460D0861\rdcp wait:406h:\rdcp update:u\r\rdcp spi:STP0=0x351E0000461BED62\rdcp wait:406h:\rdcp update:u\r\rdcp spi:STP0=0x35700000462AD263\rdcp wait:406h:\rdcp update:u\r\rdcp spi:STP0=0x35C200004639B764\rdcp wait:406h:\rdcp update:u\r\rdcp spi:STP0=0x3614000046489C65\rdcp wait:406h:\rdcp update:u\r\rdcp spi:STP0=0x3666000046578165\rdcp wait:406h:\rdcp update:u\r\rdcp spi:STP0=0x2CCCCCCD\rdcp wait:125h:\rdcp update:u\rdcp start\r")   [LabVIEW 2016]
uses:
  <vilib>/DAQmx/create/channels.llb/DAQmx Create Channel (AO-Voltage-Basic).vi
  <resource>/objmgr/daqmx.rc
  <vilib>/DAQmx/write.llb/DAQmx Write (Analog 2D DBL NChan NSamp).vi
  <vilib>/DAQmx/configure/timing.llb/DAQmx Timing (Sample Clock).vi
  <vilib>/DAQmx/configure/trigger.llb/DAQmx Start Trigger (Digital Edge).vi
panel:
  in  "source":tag
  in  "physical channels 2":tag
  in  "physical channels":tag
  in  "appended array 2":dbl[](array[numeric])=[0.85, 0.845, 0.84, 0.835, 0.83, 0.825, 0.82, 0.815, 0.8099999999999999, 0.8049999999999999, 0.8, 0.7949999999999999, 0.79, 0.785, 0.78, 0.775, 0.77, 0.765, 0.76, 0.755, 0.75, 0.7475, 0.745, 0.7425, 0.74, 0.7375, 0.735, 0.7325, 0.73, 0.7275, 0.725, 0.7225, 0.72, 0.7175, 0.715, 0.7125, 0.71, 0.7075, 0.705, 0.7025, 0.7, 0.6975, 0.6950000000000001, 0.6925, 0.6900000000000001, 0.6875, 0.685, 0.6825, 0.68, 0.6775, 0.675, 0.6725, 0.67, 0.6675, 0.665, 0.6625, 0.66, 0.6575, 0.655, 0.6525, 0.65, 0.649, 0.648, 0.647, 0.646, 0.645, 0.644, 0.643, 0.642, 0.641, 0.64, 0.639, 0.638, 0.637, 0.636, 0.635, 0.634, 0.633, 0.632, 0.631, 0.63, 0.629, 0.628, 0.627, 0.626, 0.625, 0.624, 0.623, 0.622, 0.621, 0.62, 0.619, 0.618, 0.617, 0.616, 0.615, 0.614, 0.613, 0.612, 0.611, 0.61, 0.60925, 0.6085, 0.60775, 0.607, 0.60625, 0.6054999999999999, 0.60475, 0.604, 0.60325, 0.6025, 0.60175, 0.601, 0.60025, 0.5994999999999999, 0.59875, 0.598, 0.59725, 0.5965, 0.59575, 0.595, 0.59425, 0.5934999999999999, 0.59275, 0.592, 0.5912499999999999, 0.5905, 0.58975, 0.589, 0.5882499999999999, 0.5874999999999999, 0.58675, 0.586, 0.5852499999999999, 0.5845, 0.58375, 0.583, 0.5822499999999999, 0.5814999999999999, 0.58075, 0.58, 0.57975, 0.5794999999999999, 0.5792499999999999, 0.579, 0.57875, 0.5785, 0.5782499999999999, 0.578, 0.57775, 0.5774999999999999, 0.5772499999999999, 0.577, 0.57675, 0.5765, 0.5762499999999999, 0.576, 0.57575, 0.5754999999999999, 0.5752499999999999, 0.575, 0.57475, 0.5745, 0.5742499999999999, 0.574, 0.57375, 0.5734999999999999, 0.5732499999999999, 0.573, 0.57275, 0.5725, 0.5722499999999999, 0.572, 0.57175, 0.5714999999999999, 0.5712499999999999, 0.571, 0.57075, 0.5705, 0.5702499999999999, 0.57, 0.5702499999999999, 0.5705, 0.57075, 0.571, 0.5712499999999999, 0.5714999999999999, 0.57175, 0.572, 0.5722499999999999, 0.5725, 0.57275, 0.573, 0.5732499999999999, 0.5734999999999999, 0.57375, 0.574, 0.5742499999999999, 0.5745, 0.57475, 0.575, 0.5752499999999999, 0.5754999999999999, 0.57575, 0.576, 0.5762499999999999, 0.5765, 0.57675, 0.577, 0.5772499999999999, 0.5774999999999999, 0.57775, 0.578, 0.5782499999999999, 0.5785, 0.57875, 0.579, 0.5792499999999999, 0.5794999999999999, 0.57975, 0.58, 0.58075, 0.5814999999999999, 0.5822499999999999, 0.583, 0.58375, 0.5845, 0.5852499999999999, 0.586, 0.58675, 0.5874999999999999, 0.5882499999999999, 0.589, 0.58975, 0.5905, 0.5912499999999999, 0.592, 0.59275, 0.5934999999999999, 0.59425, 0.595, 0.59575, 0.5965, 0.59725, 0.598, 0.59875, 0.5994999999999999, 0.60025, 0.601, 0.60175, 0.6025, 0.60325, 0.604, 0.60475, 0.6054999999999999, 0.60625, 0.607, 0.60775, 0.6085, 0.60925, 0.61, 0.61125, 0.6125, 0.61375, 0.615, 0.61625, 0.6174999999999999, 0.61875, 0.62, 0.62125, 0.6225, 0.62375, 0.625, 0.62625, 0.6275, 0.62875, 0.63, 0.63125, 0.6325000000000001, 0.63375, 0.635, 0.63625, 0.6375, 0.63875, 0.64, 0.64125, 0.6425000000000001, 0.64375, 0.645, 0.64625, 0.6475, 0.64875, 0.65, 0.65125, 0.6525000000000001, 0.65375, 0.655, 0.65625, 0.6575, 0.6587500000000001, 0.66, 0.6607500000000001, 0.6615, 0.66225, 0.663, 0.6637500000000001, 0.6645, 0.66525, 0.666, 0.6667500000000001, 0.6675, 0.66825, 0.669, 0.66975, 0.6705, 0.67125, 0.672, 0.67275, 0.6735, 0.67425, 0.675, 0.67575, 0.6765, 0.67725, 0.6779999999999999, 0.67875, 0.6795, 0.68025, 0.6809999999999999, 0.68175, 0.6825, 0.6832499999999999, 0.6839999999999999, 0.68475, 0.6855, 0.6862499999999999, 0.6869999999999999, 0.68775, 0.6885, 0.6892499999999999, 0.69, 0.6904999999999999, 0.691, 0.6915, 0.692, 0.6924999999999999, 0.693, 0.6935, 0.694, 0.6944999999999999, 0.695, 0.6955, 0.696, 0.6964999999999999, 0.697, 0.6975, 0.698, 0.6984999999999999, 0.699, 0.6995, 0.7, 0.7004999999999999, 0.701, 0.7015, 0.702, 0.7024999999999999, 0.703, 0.7035, 0.704, 0.7044999999999999, 0.705, 0.7055, 0.706, 0.7064999999999999, 0.707, 0.7075, 0.708, 0.7084999999999999, 0.709, 0.7095, 0.71, 0.71075, 0.7115, 0.7122499999999999, 0.713, 0.71375, 0.7144999999999999, 0.7152499999999999, 0.716, 0.71675, 0.7175, 0.7182499999999999, 0.719, 0.71975, 0.7204999999999999, 0.72125, 0.722, 0.72275, 0.7235, 0.72425, 0.725, 0.72575, 0.7264999999999999, 0.72725, 0.728, 0.72875, 0.7295, 0.73025, 0.731, 0.73175, 0.7324999999999999, 0.73325, 0.734, 0.73475, 0.7355, 0.73625, 0.737, 0.73775, 0.7384999999999999, 0.73925, 0.74, 0.7435, 0.747, 0.7505, 0.754, 0.7575000000000001, 0.761, 0.7645, 0.768, 0.7715000000000001, 0.775, 0.7785, 0.782, 0.7855000000000001, 0.789, 0.7925, 0.796, 0.7995000000000001, 0.803, 0.8065]
  out "Array":dbl[](array[numeric])=[0.85, 0.845, 0.84, 0.835, 0.83, 0.825, 0.82, 0.815, 0.8099999999999999, 0.8049999999999999, 0.8, 0.7949999999999999, 0.79, 0.785, 0.78, 0.775, 0.77, 0.765, 0.76, 0.755]
  in  "Ramp offset":dbl=-1.0 format="%#_13g"
  in  "End Freq (Hz)":i32=275000000
  in  "Power scaling factor":dbl=0.0015 format="%#_13g"
  out "Freq Step (Hz)":i32=227273
  in  "Time step (ms)":dbl=0.00325 format="%#_13g"
  out "Min DDS setting":dbl=0.6715
  in  "Start Freq (Hz)":i32=175000000
  out "appended array":dbl[][](array[numeric])=[[1.0, 1.002, 1.004, 1.006, 1.008, 1.01, 1.012, 1.014, 1.016, 1.018, 1.02, 1.022, 1.024, 1.026, 1.028, 1.03, 1.032, 1.034, 1.036, 1.038, 1.04, 1.042, 1.044, 1.046, 1.048, 1.05, 1.052, 1.054, 1.056, 1.058, 1.06, 1.062, 1.064, 1.066, 1.068, 1.07, 1.072, 1.074, 1.076, 1.078, 1.08, 1.082, 1.084, 1.086, 1.088, 1.09, 1.092, 1.094, 1.096, 1.098, 1.1, 1.102, 1.104, 1.106, 1.108, 1.11, 1.112, 1.114, 1.116, 1.118, 1.12, 1.1219999999999999, 1.124, 1.126, 1.1280000000000001, 1.13, 1.1320000000000001, 1.134, 1.1360000000000001, 1.138, 1.1400000000000001, 1.142, 1.1440000000000001, 1.146, 1.148, 1.15, 1.152, 1.154, 1.156, 1.158, 1.16, 1.162, 1.164, 1.166, 1.168, 1.17, 1.172, 1.174, 1.176, 1.178, 1.18, 1.182, 1.184, 1.186, 1.188, 1.19, 1.192, 1.194, 1.196, 1.198, 1.2, 1.2, 1.2, 1.2, 1.2, 1.2, 1.2, 1.2, 1.2, 1.2, 1.2, 1.2, 1.2, 1.2, 1.2, 1.2, 1.2, 1.2, 1.2, 1.2, 1.2, 1.2, 1.2, 1.2, 1.2, 1.2, 1.2, 1.2, 1.2, 1.2, 1.2, 1.2, 1.2, 1.2, 1.2, 1.2, 1.2, 1.2, 1.2, 1.2, 1.2, 1.2, 1.2, 1.2, 1.2, 1.2, 1.2, 1.2, 1.2, 1.2, 1.2, 1.2, 1.198, 1.196, 1.194, 1.192, 1.19, 1.188, 1.186, 1.184, 1.182, 1.18, 1.178, 1.176, 1.174, 1.172, 1.17, 1.168, 1.166, 1.164, 1.162, 1.16, 1.158, 1.156, 1.154, 1.152, 1.15, 1.148, 1.146, 1.1440000000000001, 1.142, 1.1400000000000001, 1.138, 1.1360000000000001, 1.134, 1.1320000000000001, 1.13, 1.1280000000000001, 1.126, 1.124, 1.1219999999999999, 1.12, 1.118, 1.116, 1.114, 1.112, 1.11, 1.108, 1.106, 1.104, 1.102, 1.1, 1.098, 1.096, 1.094, 1.092, 1.09, 1.088, 1.086, 1.084, 1.082, 1.08, 1.078, 1.076, 1.074, 1.072, 1.07, 1.068, 1.066, 1.064, 1.062, 1.06, 1.058, 1.056, 1.054, 1.052, 1.05, 1.048, 1.046, 1.044, 1.042, 1.04, 1.038, 1.036, 1.034, 1.032, 1.03, 1.028, 1.026, 1.024, 1.022, 1.02, 1.018, 1.016, 1.014, 1.012, 1.01, 1.008, 1.006, 1.004, 1.002, 1.0], [1.0, 1.002, 1.004, 1.006, 1.008, 1.01, 1.012, 1.014, 1.016, 1.018, 1.02, 1.022, 1.024, 1.026, 1.028, 1.03, 1.032, 1.034, 1.036, 1.038, 1.04, 1.042, 1.044, 1.046, 1.048, 1.05, 1.052, 1.054, 1.056, 1.058, 1.06, 1.062, 1.064, 1.066, 1.068, 1.07, 1.072, 1.074, 1.076, 1.078, 1.08, 1.082, 1.084, 1.086, 1.088, 1.09, 1.092, 1.094, 1.096, 1.098, 1.1, 1.102, 1.104, 1.106, 1.108, 1.11, 1.112, 1.114, 1.116, 1.118, 1.12, 1.1219999999999999, 1.124, 1.126, 1.1280000000000001, 1.13, 1.1320000000000001, 1.134, 1.1360000000000001, 1.138, 1.1400000000000001, 1.142, 1.1440000000000001, 1.146, 1.148, 1.15, 1.152, 1.154, 1.156, 1.158, 1.16, 1.162, 1.164, 1.166, 1.168, 1.17, 1.172, 1.174, 1.176, 1.178, 1.18, 1.182, 1.184, 1.186, 1.188, 1.19, 1.192, 1.194, 1.196, 1.198, 1.2, 1.2, 1.2, 1.2, 1.2, 1.2, 1.2, 1.2, 1.2, 1.2, 1.2, 1.2, 1.2, 1.2, 1.2, 1.2, 1.2, 1.2, 1.2, 1.2, 1.2, 1.2, 1.2, 1.2, 1.2, 1.2, 1.2, 1.2, 1.2, 1.2, 1.2, 1.2, 1.2, 1.2, 1.2, 1.2, 1.2, 1.2, 1.2, 1.2, 1.2, 1.2, 1.2, 1.2, 1.2, 1.2, 1.2, 1.2, 1.2, 1.2, 1.2, 1.2, 1.198, 1.196, 1.194, 1.192, 1.19, 1.188, 1.186, 1.184, 1.182, 1.18, 1.178, 1.176, 1.174, 1.172, 1.17, 1.168, 1.166, 1.164, 1.162, 1.16, 1.158, 1.156, 1.154, 1.152, 1.15, 1.148, 1.146, 1.1440000000000001, 1.142, 1.1400000000000001, 1.138, 1.1360000000000001, 1.134, 1.1320000000000001, 1.13, 1.1280000000000001, 1.126, 1.124, 1.1219999999999999, 1.12, 1.118, 1.116, 1.114, 1.112, 1.11, 1.108, 1.106, 1.104, 1.102, 1.1, 1.098, 1.096, 1.094, 1.092, 1.09, 1.088, 1.086, 1.084, 1.082, 1.08, 1.078, 1.076, 1.074, 1.072, 1.07, 1.068, 1.066, 1.064, 1.062, 1.06, 1.058, 1.056, 1.054, 1.052, 1.05, 1.048, 1.046, 1.044, 1.042, 1.04, 1.038, 1.036, 1.034, 1.032, 1.03, 1.028, 1.026, 1.024, 1.022, 1.02, 1.018, 1.016, 1.014, 1.012, 1.01, 1.008, 1.006, 1.004, 1.002, 1.0]]
  in  "Plateau duration (ms)":dbl=1.0
  in  "Ramp duration (ms)":dbl=2.0
  in  "No of samples in ramp":dbl=100.0
  in  "Ramp Amplitude (V)}":dbl=0.2
  in  "error in":errorcluster
  out "Array 2":i32[](array[numeric])=[175000000, 175227273, 175454545, 175681818, 175909091, 176136364, 176363636, 176590909, 176818182, 177045455, 177272727, 177500000, 177727273, 177954545, 178181818, 178409091, 178636364, 178863636, 179090909, 179318182, 179545455, 179772727, 180000000, 180227273, 180454545, 180681818, 180909091, 181136364, 181363636, 181590909, 181818182, 182045455, 182272727, 182500000, 182727273, 182954545, 183181818, 183409091, 183636364, 183863636, 184090909, 184318182, 184545455, 184772727, 185000000, 185227273, 185454545, 185681818, 185909091, 186136364, 186363636, 186590909, 186818182, 187045455, 187272727, 187500000, 187727273, 187954545, 188181818, 188409091, 188636364, 188863636, 189090909, 189318182, 189545455, 189772727, 190000000, 190227273, 190454545, 190681818, 190909091, 191136364, 191363636, 191590909, 191818182, 192045455, 192272727, 192500000, 192727273, 192954545, 193181818, 193409091, 193636364, 193863636, 194090909, 194318182, 194545455, 194772727, 195000000, 195227273, 195454545, 195681818, 195909091, 196136364, 196363636, 196590909, 196818182, 197045455, 197272727, 197500000, 197727273, 197954545, 198181818, 198409091, 198636364, 198863636, 199090909, 199318182, 199545455, 199772727, 200000000, 200227273, 200454545, 200681818, 200909091, 201136364, 201363636, 201590909, 201818182, 202045455, 202272727, 202500000, 202727273, 202954545, 203181818, 203409091, 203636364, 203863636, 204090909, 204318182, 204545455, 204772727, 205000000, 205227273, 205454545, 205681818, 205909091, 206136364, 206363636, 206590909, 206818182, 207045455, 207272727, 207500000, 207727273, 207954545, 208181818, 208409091, 208636364, 208863636, 209090909, 209318182, 209545455, 209772727, 210000000, 210227273, 210454545, 210681818, 210909091, 211136364, 211363636, 211590909, 211818182, 212045455, 212272727, 212500000, 212727273, 212954545, 213181818, 213409091, 213636364, 213863636, 214090909, 214318182, 214545455, 214772727, 215000000, 215227273, 215454545, 215681818, 215909091, 216136364, 216363636, 216590909, 216818182, 217045455, 217272727, 217500000, 217727273, 217954545, 218181818, 218409091, 218636364, 218863636, 219090909, 219318182, 219545455, 219772727, 220000000, 220227273, 220454545, 220681818, 220909091, 221136364, 221363636, 221590909, 221818182, 222045455, 222272727, 222500000, 222727273, 222954545, 223181818, 223409091, 223636364, 223863636, 224090909, 224318182, 224545455, 224772727, 225000000, 225227273, 225454545, 225681818, 225909091, 226136364, 226363636, 226590909, 226818182, 227045455, 227272727, 227500000, 227727273, 227954545, 228181818, 228409091, 228636364, 228863636, 229090909, 229318182, 229545455, 229772727, 230000000, 230227273, 230454545, 230681818, 230909091, 231136364, 231363636, 231590909, 231818182, 232045455, 232272727, 232500000, 232727273, 232954545, 233181818, 233409091, 233636364, 233863636, 234090909, 234318182, 234545455, 234772727, 235000000, 235227273, 235454545, 235681818, 235909091, 236136364, 236363636, 236590909, 236818182, 237045455, 237272727, 237500000, 237727273, 237954545, 238181818, 238409091, 238636364, 238863636, 239090909, 239318182, 239545455, 239772727, 240000000, 240227273, 240454545, 240681818, 240909091, 241136364, 241363636, 241590909, 241818182, 242045455, 242272727, 242500000, 242727273, 242954545, 243181818, 243409091, 243636364, 243863636, 244090909, 244318182, 244545455, 244772727, 245000000, 245227273, 245454545, 245681818, 245909091, 246136364, 246363636, 246590909, 246818182, 247045455, 247272727, 247500000, 247727273, 247954545, 248181818, 248409091, 248636364, 248863636, 249090909, 249318182, 249545455, 249772727, 250000000, 250227273, 250454545, 250681818, 250909091, 251136364, 251363636, 251590909, 251818182, 252045455, 252272727, 252500000, 252727273, 252954545, 253181818, 253409091, 253636364, 253863636, 254090909, 254318182, 254545455, 254772727, 255000000, 255227273, 255454545, 255681818, 255909091, 256136364, 256363636, 256590909, 256818182, 257045455, 257272727, 257500000, 257727273, 257954545, 258181818, 258409091, 258636364, 258863636, 259090909, 259318182, 259545455, 259772727, 260000000, 260227273, 260454545, 260681818, 260909091, 261136364, 261363636, 261590909, 261818182, 262045455, 262272727, 262500000, 262727273, 262954545, 263181818, 263409091, 263636364, 263863636, 264090909, 264318182, 264545455, 264772727, 265000000, 265227273, 265454545, 265681818, 265909091, 266136364, 266363636, 266590909, 266818182, 267045455, 267272727, 267500000, 267727273, 267954545, 268181818, 268409091, 268636364, 268863636, 269090909, 269318182, 269545455, 269772727, 270000000, 270227273, 270454545, 270681818, 270909091, 271136364, 271363636, 271590909, 271818182, 272045455, 272272727, 272500000, 272727273, 272954545, 273181818, 273409091, 273636364, 273863636, 274090909, 274318182, 274545455, 274772727]
  out "return count":u32=26996
  out "error out":errorcluster={"status"=TRUE, "code"=-1073807339, "source"="VISA Read in DDSSequence_STPrampv1.vi"}
  out "read buffer":string
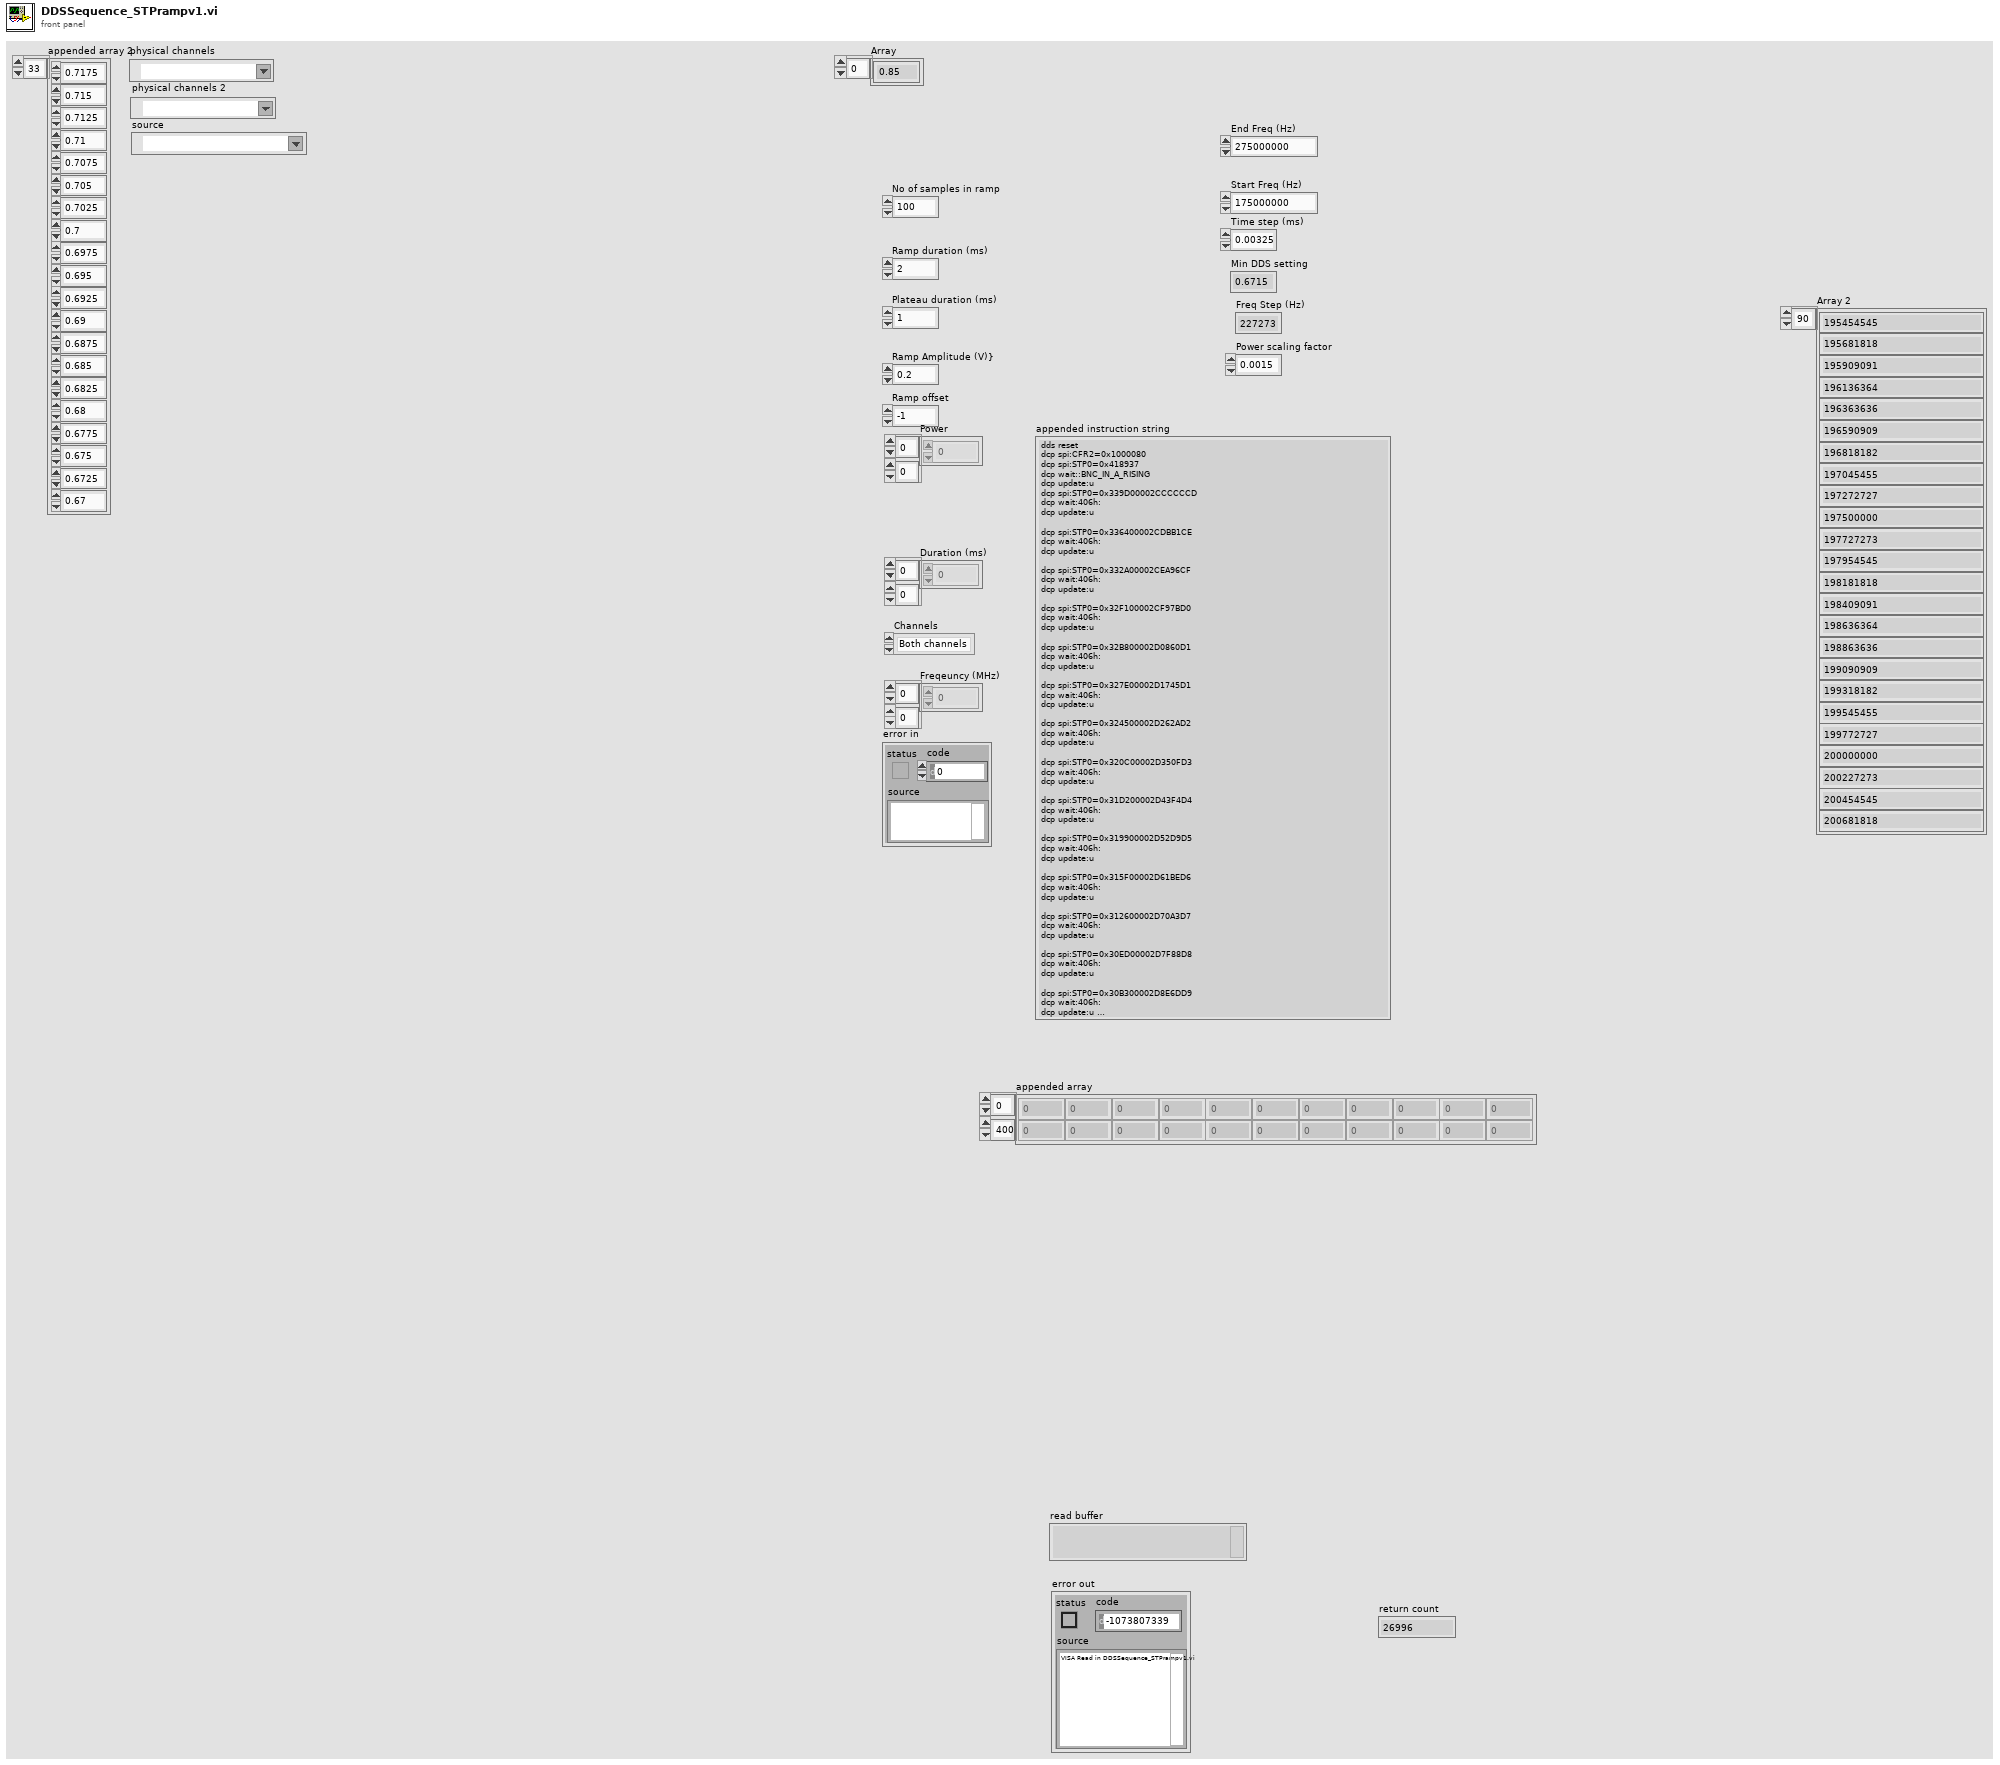
[diagram p1: front panel]
types:
  T1 = enum32{"Channel 0", "Channel 1", "Both channels"}
  T2 = enum32{"O_RAMP_SWP_OVR", "RAM_SWP_OVR", "O_DROVER", "DROVER", "O_SPI_FIFO_EV1", "SPI_FIFO_EV1", "O_SPI_FIFO_EV0", "SPI_FIFO_EV0", "O_SPI_FIFO_FLUSHED", "SPI_FIFO_FLUSHED", "BNC_IN_B_LEVEL", "BNC_IN_B_FALLING", "BNC_IN_B_RISING", "BNC_IN_A_LEVEL", "BNC_IN_A_FALLING", "BNC_IN_A_RISING", "ALL_SPI_FIFOS_FLUSHED", "NONE"}
  T3 = cluster{"Enable ASF from STP (F)":bool, "Digital ramp enable (F)":bool, "Digital ramp no-dwell high (F)":bool, "Digital ramp no-dwell low (F)":bool, "Matched latency enable (T)":bool, "Parallel data port enable (F)":bool}
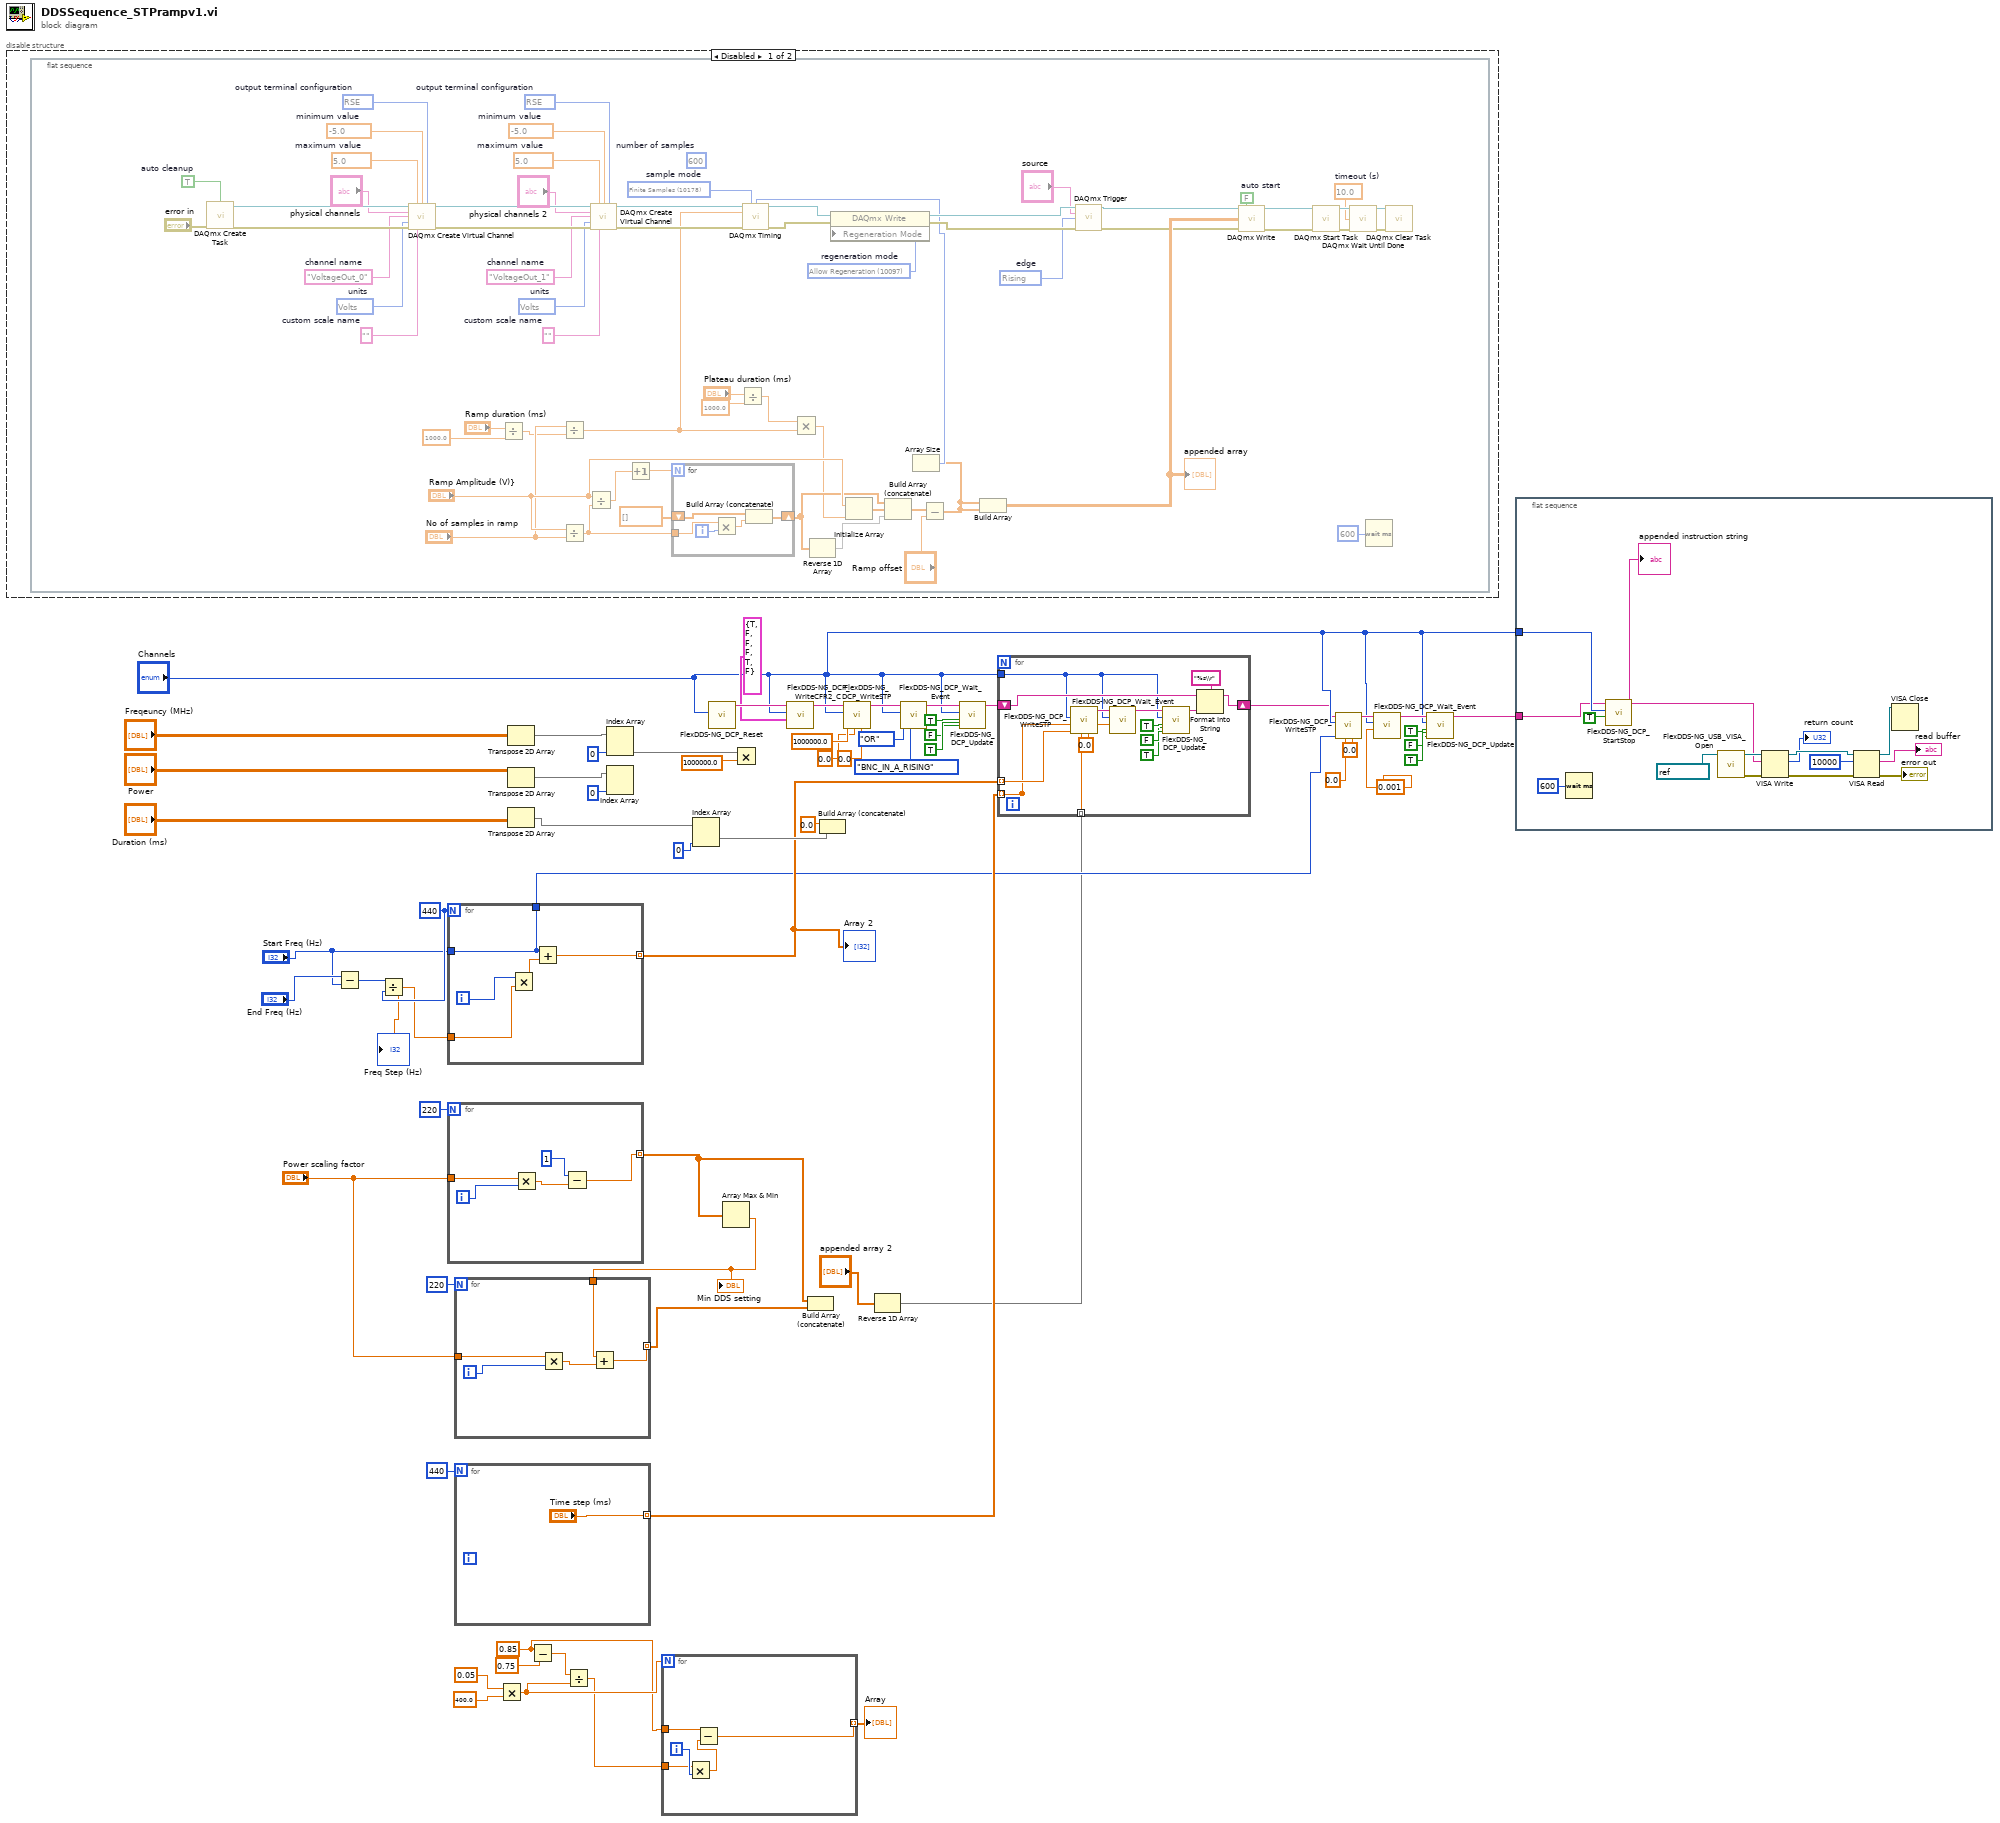
[diagram p0: block diagram]
diagram:
  w5 = 0.85 ("x")
  w14 = 440
  n1 = disable-structure shown="Disabled" {
    frame Disabled {
      n2 = flat-sequence {
        frame #0 {
          w92 = 10280 items=["Rising"=10280, "Falling"=10171]  # edge
          w94 = 10097 items=["Allow Regeneration"=10097, "Do Not Allow Regeneration"=10158]  # regeneration mode
          w97 = 10178 items=["Finite Samples"=10178, "Continuous Samples"=10123, "Hardware Timed Single Point"=12522]  # sample mode
          (unwired) 600  # number of samples
          w100 = 10083 items=["Default"=-1, "RSE"=10083, "Differential"=10106, "Pseudodifferential"=12529]  # output terminal configuration
          w101 = 10348 items=["Volts"=10348, "From Custom Scale"=10065]  # units
          w102 = "VoltageOut_1"  # channel name
          w104 = ""  # custom scale name
          w105 = -5.0  # minimum value
          w106 = 5.0  # maximum value
          w108 = 10083 items=["Default"=-1, "RSE"=10083, "Differential"=10106, "Pseudodifferential"=12529]  # output terminal configuration
          w109 = 10348 items=["Volts"=10348, "From Custom Scale"=10065]  # units
          w110 = "VoltageOut_0"  # channel name
          w112 = ""  # custom scale name
          w113 = -5.0  # minimum value
          w114 = 5.0  # maximum value
          w116 = TRUE  # auto cleanup
          w122 = 10.0  # timeout (s)
          w126 = FALSE  # auto start
          n3 = call <vilib>:"DAQmx Create Task.vi"("auto cleanup"=w116, "error in"="error in") -> ("task out"=w115:refnum<k21>, "error out"=w117:errorcluster)  [unwired: 12 in]
          n4 = call-poly <vilib>:"DAQmx Create Virtual Channel.vi"("task in"=w115, "maximum value"=w114, "minimum value"=w113, "output terminal configuration"=w108, "physical channels"="physical channels", "name to assign"=w110, "units"=w109, "error in"=w117, "custom scale name"=w112) -> ("task out"=w107:refnum<k21>, "error out"=w111:errorcluster)  [unwired: 5 in]
          n5 = Divide(x="Ramp duration (ms)", y=1000.0) -> (x/y=w79:dbl)
          n6 = Divide(x="No of samples in ramp", y=w79) -> (x/y=w74:dbl)
          n7 = Divide(x="Ramp Amplitude (V)}", y="No of samples in ramp") -> (x/y=w90:dbl)
          n8 = Divide(x="Ramp Amplitude (V)}", y=w90) -> (x/y=w89:dbl)
          n9 = call-poly <vilib>:"DAQmx Create Virtual Channel.vi"("task in"=w107, "maximum value"=w106, "minimum value"=w105, "output terminal configuration"=w100, "physical channels"="physical channels 2", "name to assign"=w102, "units"=w101, "error in"=w111, "custom scale name"=w104) -> ("task out"=w98:refnum<k21>, "error out"=w103:errorcluster)  [unwired: 5 in]
          n10 = Increment(x=w89) -> (x+1=w88:dbl)
          n11 = for {
            N: w88 -> [_]
            shift-right: [w129] -> w86
            shift-left: dbl[] [] -> [w128]
            tunnel: w90 -> [w127]
            i -> [w131]
            n12 = Multiply(x=w127, y=w131) -> (x*y=w130:dbl)
            n13 = Build Array (concatenate)(w128, w130) -> (w129:dbl[])
          }
          n14 = Divide(x="Plateau duration (ms)", y=1000.0) -> (x/y=w73:dbl)
          n15 = Multiply(x=w73, y=w74) -> (x*y=w72:dbl)
          n16 = Reverse 1D Array(array=w86) -> (reversed array=w84:dbl[])
          n17 = Initialize Array("Ramp Amplitude (V)}", w72) -> (w85:dbl[])
          n18 = Build Array (concatenate)(w86, w85, w84) -> (w69:dbl[])
          n19 = Subtract(x=w69, y="Ramp offset") -> (x-y=w68:dbl[])
          n20 = Array Size(array=w68) -> (size(s)=w71:i32)
          n21 = call-poly <vilib>:"DAQmx Timing.vi"("task/channels in"=w98, "sample mode"=w97, "samples per channel"=w71, "rate"=w74, "error in"=w103) -> ("task out"=w96:refnum<k21>, "error out"=w99:errorcluster)  [unwired: 9 in]
          n22 = property class="DAQmx Write"(reference=w96, error in=w99, "Regeneration Mode"=w94) -> (reference out=w93:refnum<k21>, error out=w95:errorcluster)
          n23 = Build Array(w68, w68) -> (w83:dbl[][])
          "appended array" <- w83
          n24 = call-poly <vilib>:"DAQmx Trigger.vi"("task/channels in"=w93, "source"="source", "edge"=w92, "error in"=w95) -> ("task out"=w78:refnum<k21>, "error out"=w77:errorcluster)  [unwired: 10 in]
          n25 = call-poly <vilib>:"DAQmx Write.vi"("task/channels in"=w78, "auto start"=w126, "data"=w83, "error in"=w77) -> ("task out"=w121:refnum<k21>, "error out"=w120:errorcluster)  [unwired: 9 in, 1 out]
          n26 = call <vilib>:"DAQmx Start Task.vi"("task/channels in"=w121, "error in"=w120) -> ("task out"=w125:refnum<k21>, "error out"=w124:errorcluster)  [unwired: 12 in]
          n27 = call <vilib>:"DAQmx Wait Until Done.vi"("task/channels in"=w125, "timeout (sec)"=w122, "error in"=w124) -> ("task out"=w119:refnum<k21>, "error out"=w123:errorcluster)  [unwired: 11 in]
          n28 = Wait (ms)(milliseconds to wait=u32 600) -> ()  [unwired: 1 out]
          n29 = call <vilib>:"DAQmx Clear Task.vi"("task in"=w119, "error in"=w123) -> ()  [unwired: 13 in, 1 out]
        }
      }
    }
    frame Enabled {
    }
  }
  n30 = Subtract(x="End Freq (Hz)", y="Start Freq (Hz)") -> (x-y=w15:i32)
  n31 = Divide(x=w15, y=w14) -> (x/y=w13:dbl)
  "Freq Step (Hz)" <- w13
  n32 = for {
    N: w14 -> [_]
    tunnel: [w134] -> w22 mode=indexing
    tunnel: [w133] -> w17
    tunnel: "Start Freq (Hz)" -> [w133]
    tunnel: w13 -> [w132]
    i -> [w136]
    n33 = Multiply(x=w136, y=w132) -> (x*y=w135:dbl)
    n34 = Add(x=w133, y=w135) -> (x+y=w134:dbl)
  }
  "Array 2" <- w22
  n35 = for {
    N: 220 -> [_]
    tunnel: [w138] -> w20 mode=indexing
    tunnel: "Power scaling factor" -> [w137]
    i -> [w140]
    n36 = Multiply(x=w137, y=w140) -> (x*y=w139:dbl)
    n37 = Subtract(x=1 ("y"), y=w139) -> (x-y=w138:dbl)
  }
  n38 = for {
    N: 440 -> [_]
    tunnel: ["Time step (ms)"] -> w34 mode=indexing
  }
  n39 = Multiply(x=0.05, y=400.0) -> (x*y=w6:dbl)
  n40 = Transpose 2D Array(2D array="Freqeuncy (MHz)") -> (transposed array=w56:dbl[][])
  n41 = Transpose 2D Array(2D array="Power") -> (transposed array=w54:dbl[][])
  n42 = Transpose 2D Array(2D array="Duration (ms)") -> (transposed array=w63:dbl[][])
  n43 = Subtract(x=w5, y=0.75) -> (x-y=w7:dbl)
  n44 = Divide(x=w7, y=w6) -> (x/y=w4:dbl)
  n45 = Index Array(array=w56, index (col)=0 ("index (row)")) -> (element=w58:dbl[])  [unwired: 1 in]
  n46 = Index Array(array=w54, index (col)=0 ("index (row)")) -> ()  [unwired: 1 in, 1 out]
  n47 = for {
    N: w6 -> [_]
    tunnel: w5 -> [w147]
    tunnel: w4 -> [w145]
    tunnel: [w143] -> w3 mode=indexing
    i -> [w146]
    n48 = Multiply(x=w145, y=w146) -> (x*y=w144:dbl)
    n49 = Subtract(x=w147, y=w144) -> (x-y=w143:dbl)
  }
  "Array" <- w3
  n50 = Index Array(array=w63, index (col)=0 ("index (row)")) -> (element=w61:dbl[])  [unwired: 1 in]
  n51 = call "FlexDDS-NG_DCP_Reset.vi"("Channels"="Channels") -> ("appended instruction string"=w41:string)  [unwired: 10 in]
  n52 = Array Max & Min(array=w20) -> (min value=w18:dbl)  [unwired: 3 out]
  "Min DDS setting" <- w18
  n53 = for {
    N: 220 -> [_]
    tunnel: [w150] -> w19 mode=indexing
    tunnel: w18 -> [w149]
    tunnel: "Power scaling factor" -> [w148]
    i -> [w151]
    n54 = Multiply(x=w148, y=w151) -> (x*y=w152:dbl)
    n55 = Add(x=w149, y=w152) -> (x+y=w150:dbl)
  }
  n56 = Multiply(x=w58, y=1000000.0 ("frequency Hz (0..400M)")) -> ()  [unwired: 1 out]
  n57 = call "FlexDDS-NG_DCP_WriteCFR2_C.vi"("CFR2 bits"=T3 {"Enable ASF from STP (F)"=TRUE, "Digital ramp enable (F)"=FALSE, "Digital ramp no-dwell high (F)"=FALSE, "Digital ramp no-dwell low (F)"=FALSE, "Matched latency enable (T)"=TRUE, "Parallel data port enable (F)"=FALSE} ("CFR2 bits 2"), "Channels"="Channels", "initial instruction string"=w41) -> ("appended instruction string"=w40:string)  [unwired: 8 in]
  n58 = Build Array (concatenate)(w20, w19) -> ()  [unwired: 1 out]
  n59 = Build Array (concatenate)(0.0 ("phase degrees (0..360)"), w61) -> ()  [unwired: 1 out]
  n60 = call "FlexDDS-NG_DCP_WriteSTP.vi"("phase degrees (0..360)"=0.0, "amplitude (0..1)"=0.0, "frequency Hz (0..400M)"=1000000.0, "Channels"="Channels", "initial instruction string"=w40) -> ("appended instruction string"=w46:string)  [unwired: 6 in]
  n61 = Reverse 1D Array(array="appended array 2") -> (reversed array=w2:dbl[])
  n62 = call "FlexDDS-NG_DCP_Wait_Event.vi"("Event 1"=T2."BNC_IN_A_RISING", "AND/OR"=enum32{"AND", "OR"}."OR", "Channels in"="Channels", "appended instruction string in"=w46) -> ("appended instruction string"=w45:string)  [unwired: 7 in]
  n63 = call "FlexDDS-NG_DCP_Update.vi"("ONLY IO_UPDATE"=TRUE, "DRCTL(true=+, false=-)"=FALSE ("DRCTL(true=+, false=-) 2"), "IO_UPDATE(true=u, false = '')"=TRUE ("IO_UPDATE(true=u, false = '')  2"), "Channels"="Channels", "appended instruction string in"=w45) -> ("appended instruction string out"=w50:string)  [unwired: 6 in]
  n64 = for {
    shift-right: [w158] -> w24
    shift-left: w50 -> [w159]
    tunnel: "Channels" -> [w156]
    tunnel: w34 -> [w154] mode=indexing
    tunnel: w22 -> [w155] mode=indexing
    tunnel: [w154] -> _ mode=indexing
    tunnel: w2 -> [w153] mode=indexing
    n65 = call "FlexDDS-NG_DCP_WriteSTP.vi"("phase degrees (0..360)"=0.0, "amplitude (0..1)"=w153, "frequency Hz (0..400M)"=w155, "Channels"=w156) -> ("appended instruction string"=w161:string)  [unwired: 7 in]
    n66 = call "FlexDDS-NG_DCP_Wait_Event.vi"("waiting time [ms]"=w154, "Channels in"=w156, "appended instruction string in"=w161) -> ("appended instruction string"=w162:string)  [unwired: 8 in]
    n67 = call "FlexDDS-NG_DCP_Update.vi"("ONLY IO_UPDATE"=TRUE, "DRCTL(true=+, false=-)"=FALSE ("DRCTL(true=+, false=-) 2"), "IO_UPDATE(true=u, false = '')"=TRUE ("IO_UPDATE(true=u, false = '')  2"), "Channels"=w156, "appended instruction string in"=w162) -> ("appended instruction string out"=w157:string)  [unwired: 6 in]
    n68 = Format Into String(format string="%s\\r", initial string=w159, w157) -> (resulting string=w158:string)  [unwired: 1 in, 1 out]
  }
  n69 = call "FlexDDS-NG_DCP_WriteSTP.vi"("phase degrees (0..360)"=0.0, "amplitude (0..1)"=0.0, "frequency Hz (0..400M)"=w17, "Channels"="Channels", "initial instruction string"=w24) -> ("appended instruction string"=w33:string)  [unwired: 6 in]
  n70 = call "FlexDDS-NG_DCP_Wait_Event.vi"("waiting time [ms]"=0.001, "Channels in"="Channels", "appended instruction string in"=w33) -> ("appended instruction string"=w32:string)  [unwired: 8 in]
  n71 = call "FlexDDS-NG_DCP_Update.vi"("ONLY IO_UPDATE"=TRUE, "DRCTL(true=+, false=-)"=FALSE ("DRCTL(true=+, false=-) 2"), "IO_UPDATE(true=u, false = '')"=TRUE ("IO_UPDATE(true=u, false = '')  2"), "Channels"="Channels", "appended instruction string in"=w32) -> ("appended instruction string out"=w23:string)  [unwired: 6 in]
  n72 = flat-sequence {
    tunnel: "Channels" -> [w169]
    tunnel: w23 -> [w168]
    frame #0 {
      n73 = Wait (ms)(milliseconds to wait=u32 600) -> ()  [unwired: 1 out]
      n74 = call "FlexDDS-NG_DCP_StartStop.vi"("start (T) stop (F)"=TRUE, "Channels"=w169, "initial instruction string"=w168) -> ("appended instruction string"=w170:string)  [unwired: 8 in]
      "appended instruction string" <- w170
      n75 = call "FlexDDS-NG_USB_VISA_Open.vi"("FlexDDS-NG USB VISA resource name (COM)"=refnum<visa-resource-name> "COM7") -> ("error out"=w172:errorcluster, "FlexDDS-NG USB VISA resource name out"=w173:refnum<visa-resource-name>)  [unwired: 9 in]
      n76 = VISA Write(VISA resource name=w173, write buffer=w170, error in (no error)=w172) -> (VISA resource name out=w177:refnum<visa-resource-name>, return count=→"return count":u32, error out=w175:errorcluster)
      n77 = VISA Read(VISA resource name=w177, byte count=u32 10000, error in (no error)=w175) -> (VISA resource name out=w180:refnum<visa-resource-name>, read buffer=→"read buffer":string, error out=→"error out":errorcluster)  [unwired: 1 out]
      n78 = VISA Close(VISA resource name=w180) -> ()  [unwired: 1 in, 1 out]
    }
  }
